vi "LC-MISDK_UserCalibration.vi"() -> ()   [LabVIEW 2015]
uses:
  C:/Users/e09031/Documents/GMA/LC-160/Labview/Sample_LC-MISDK/LC-MISDK.dll
  LC-MISDK.dll
panel:
  in  "タイムスタンプ":timestamp
  out "CalError":dbl
  out "error out":errorcluster caption="エラー出力"
  out "ErrorCode":dbl
  in  "Before_B 2":bool
  in  "Before_G 2":bool
  in  "Before_R 2":bool
  in  "Before_W 2":bool
  in  "After_B":T1
  in  "After_G":T2
  in  "After_R":T3
  in  "After_W":T4
  in  "Before_B":T5
  in  "Before_G":T6
  in  "Before_R":T7
  in  "Before_W":T8
  out "Error Message":string
  in  "EXIT":bool
  in  "Calib":bool
  in  "ID":string
  in  "Color Space":T9(ring)
  in  "Calib.Ch":T10(ring)
  in  "Type of Calibration":enum32{"Single-Point", "RGB", "WRGB"}(radio)
  # "Value before Calibration"
  # "Value after Calibration"
  # "X"
  # "Y"
  # "Z"
  # "X"
  # "Y"
  # "Z"
  # "White"
  # "White"
  # "Red"
  # "Red"
  # "Green"
  # "Green"
  # "Blue"
  # "Blue"
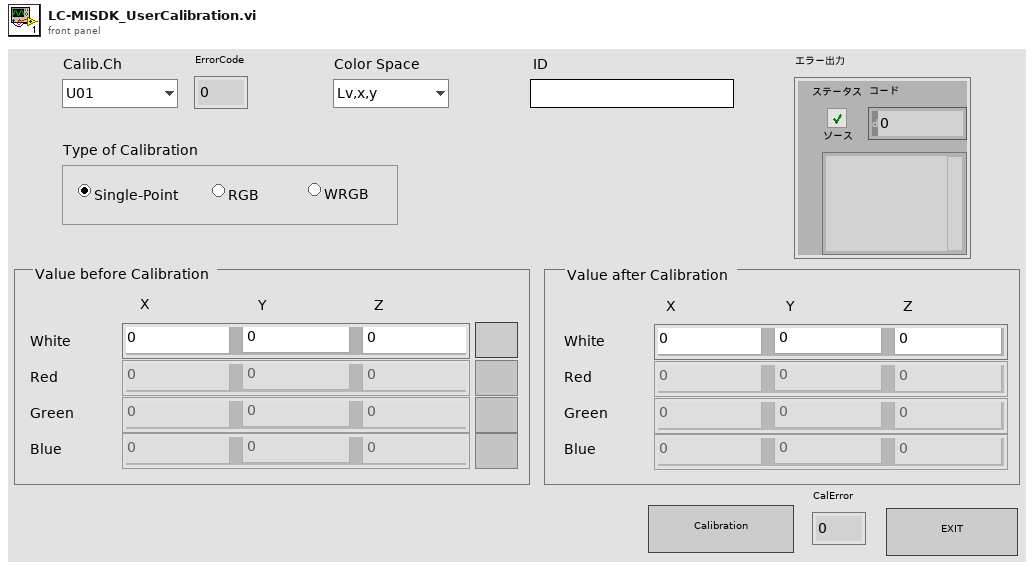
[diagram p1: front panel]
types:
  T1 = cluster{"After_B1":dbl, "After_B2":dbl, "After_B3":dbl}
  T2 = cluster{"After_G1":dbl, "After_G2":dbl, "After_G3":dbl}
  T3 = cluster{"After_R1":dbl, "After_R2":dbl, "After_R3":dbl}
  T4 = cluster{"After_W1":dbl, "After_W2":dbl, "After_W3":dbl}
  T5 = cluster{"before_B1":dbl, "Before_B2":dbl, "Before_B3":dbl}
  T6 = cluster{"before_G1":dbl, "Before_G2":dbl, "Before_G3":dbl}
  T7 = cluster{"before_R1":dbl, "Before_R2":dbl, "Before_R3":dbl}
  T8 = cluster{"before_W1":dbl, "Before_W2":dbl, "Before_W3":dbl}
  T9 = enum16{"Lv,x,y", "Lv,u',v'", "Lv,Tcp,duv", "X,Y,Z", "Lv,λd,Pe"}
  T10 = enum16{"U01", "U02", "U03", "U04", "U05", "U06", "U07", "U08", "U09", "U10"}
  T11 = cluster{"get_Item":dbl, "get_Item":dbl, "get_Item":dbl}
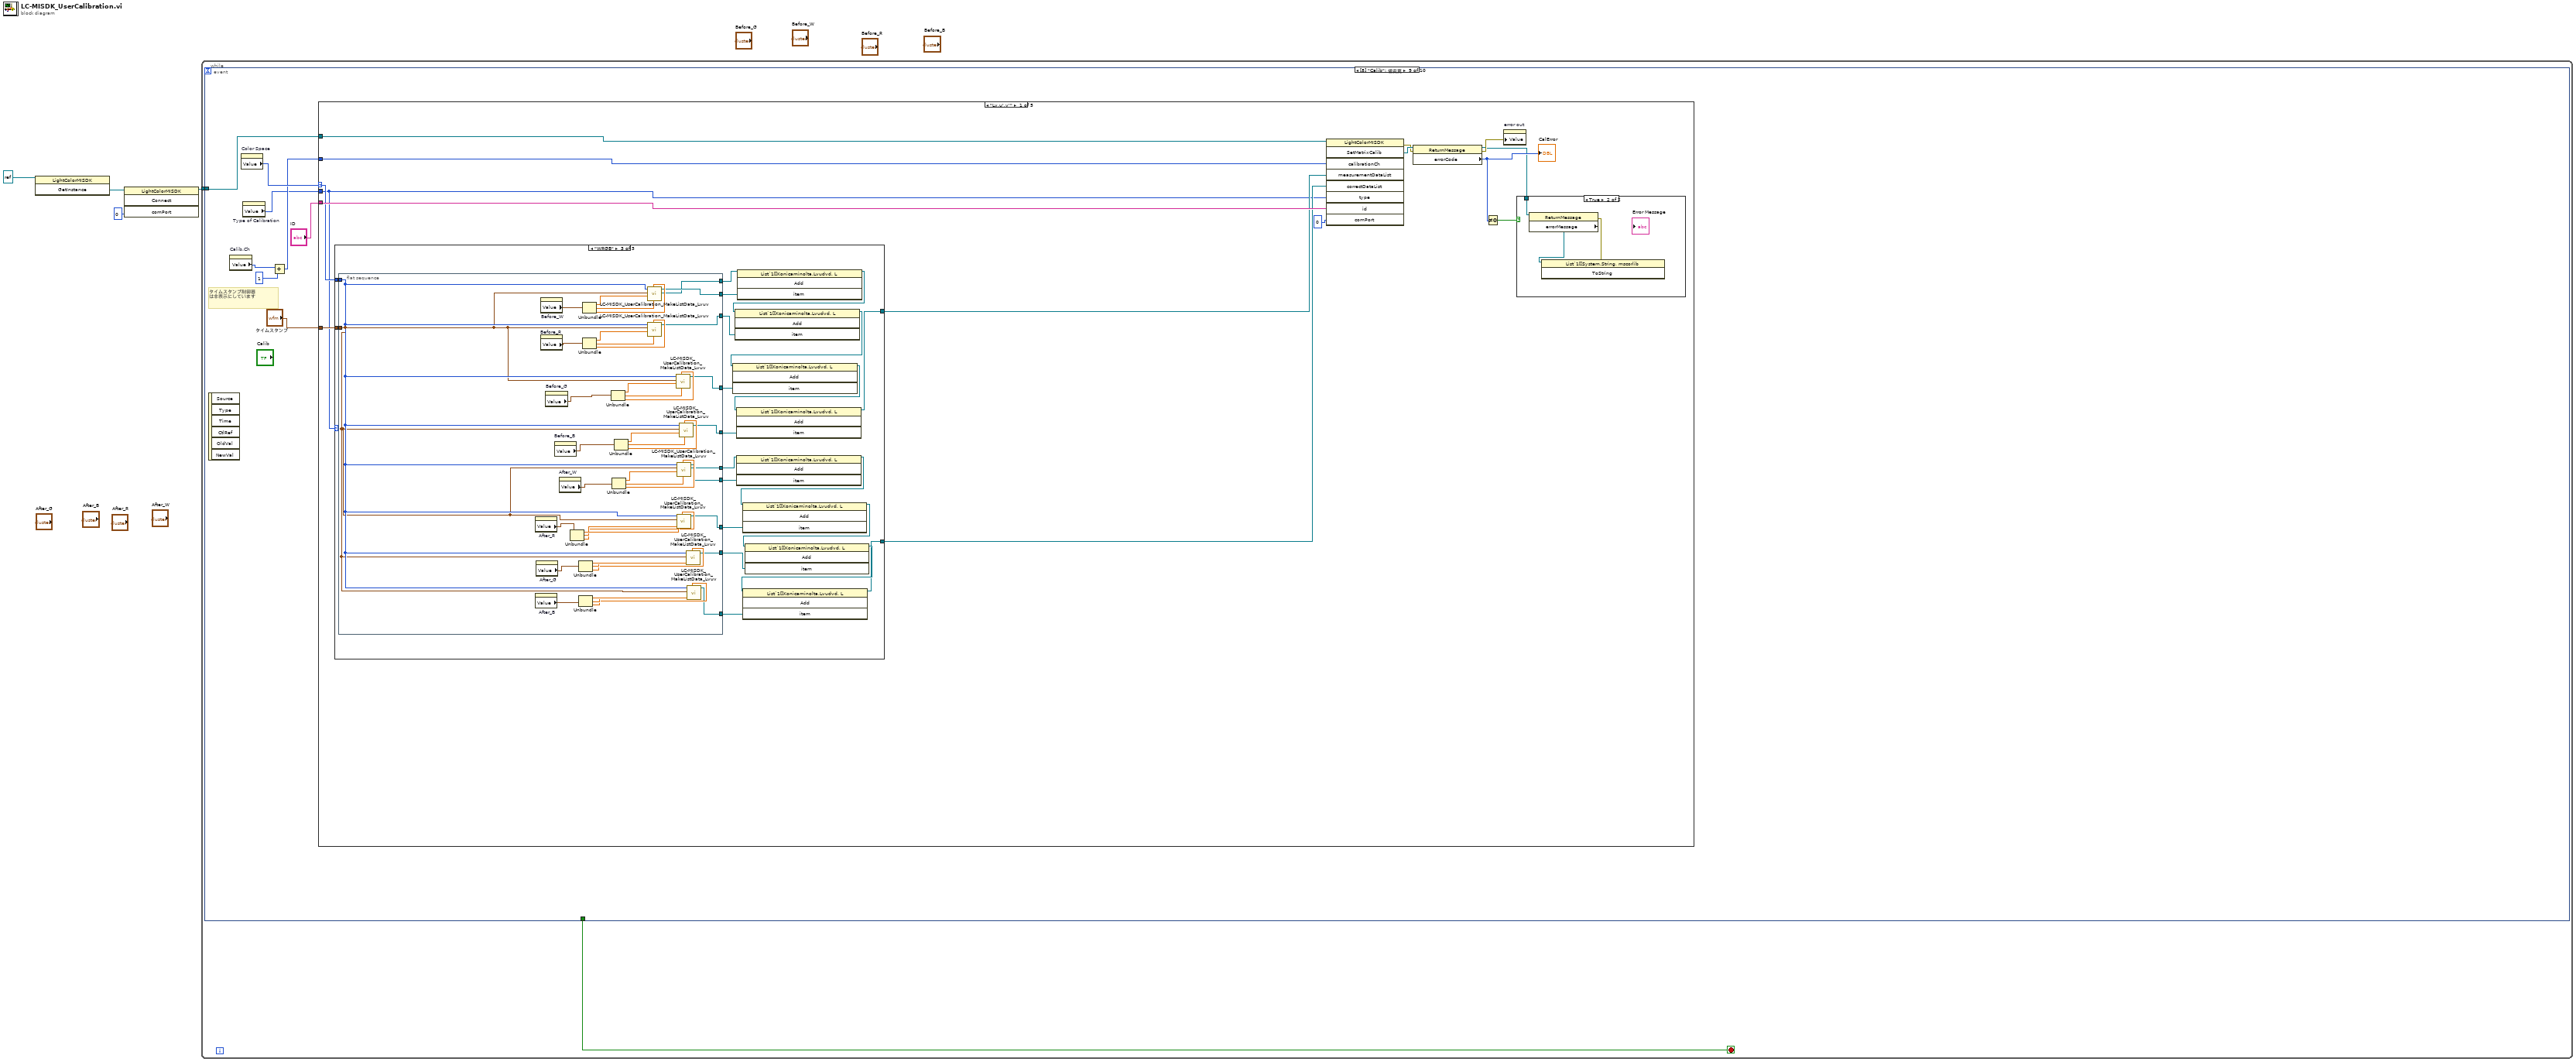
[diagram p0: block diagram]
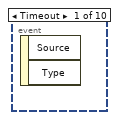
[diagram p2: hidden frame]
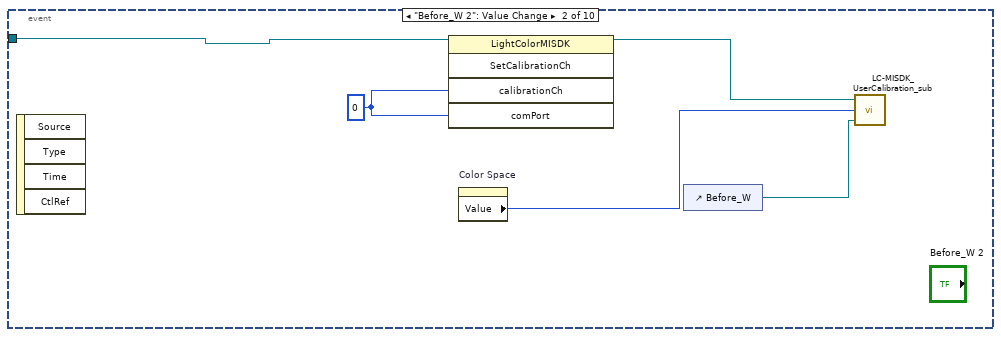
[diagram p3: hidden frame]
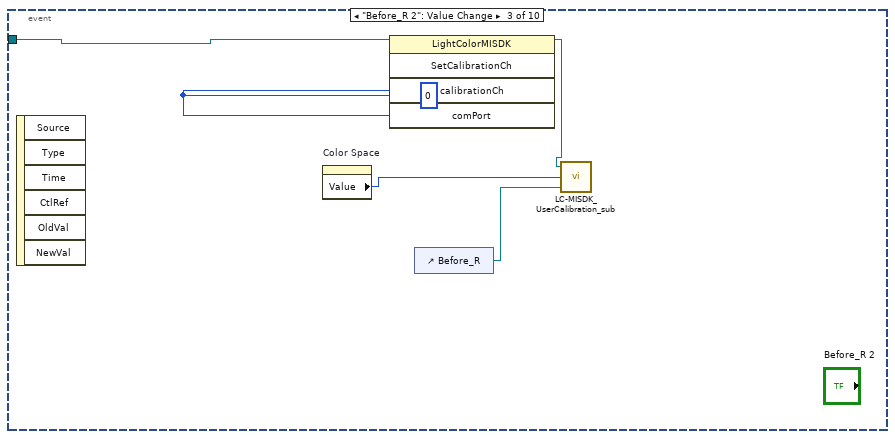
[diagram p4: hidden frame]
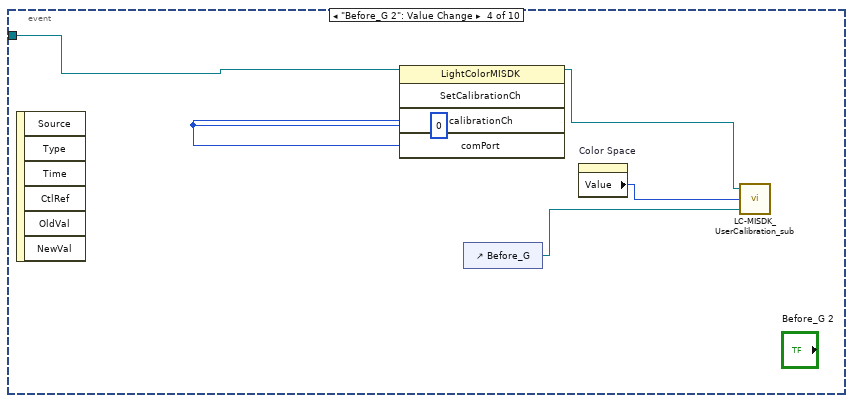
[diagram p5: hidden frame]
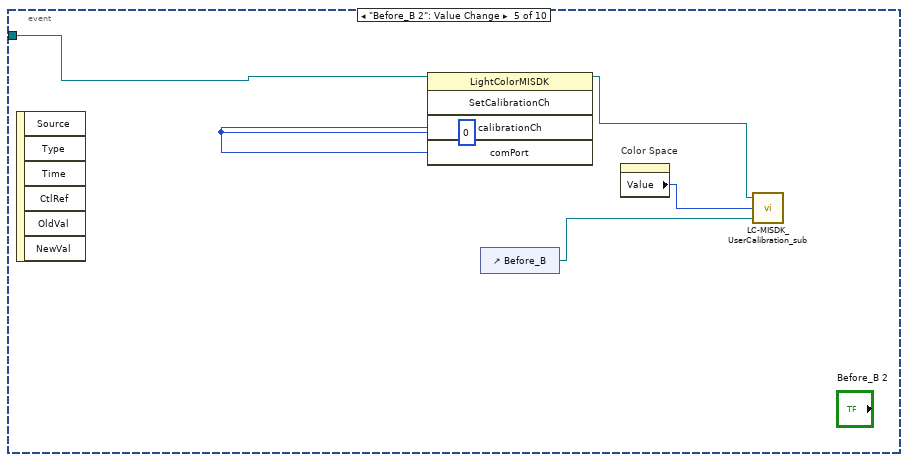
[diagram p6: hidden frame]
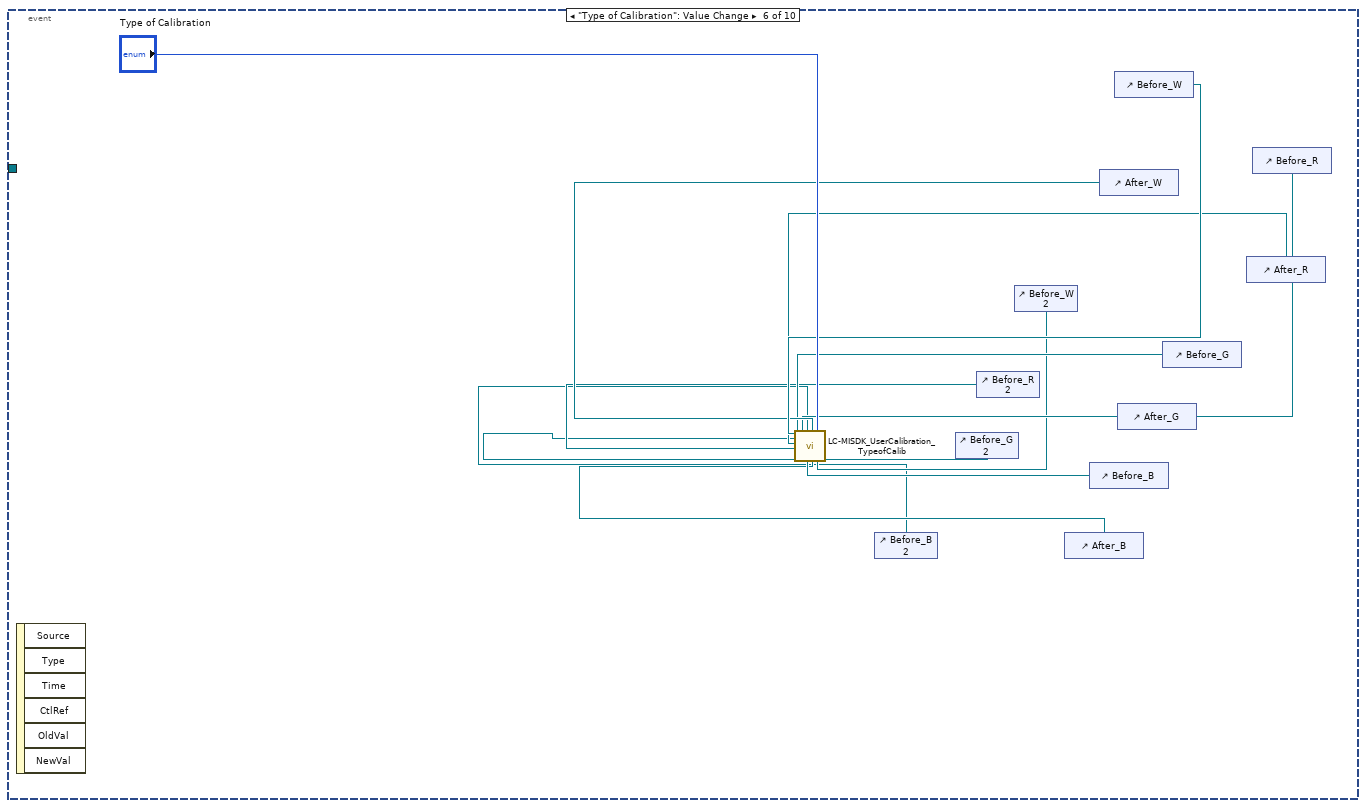
[diagram p7: hidden frame]
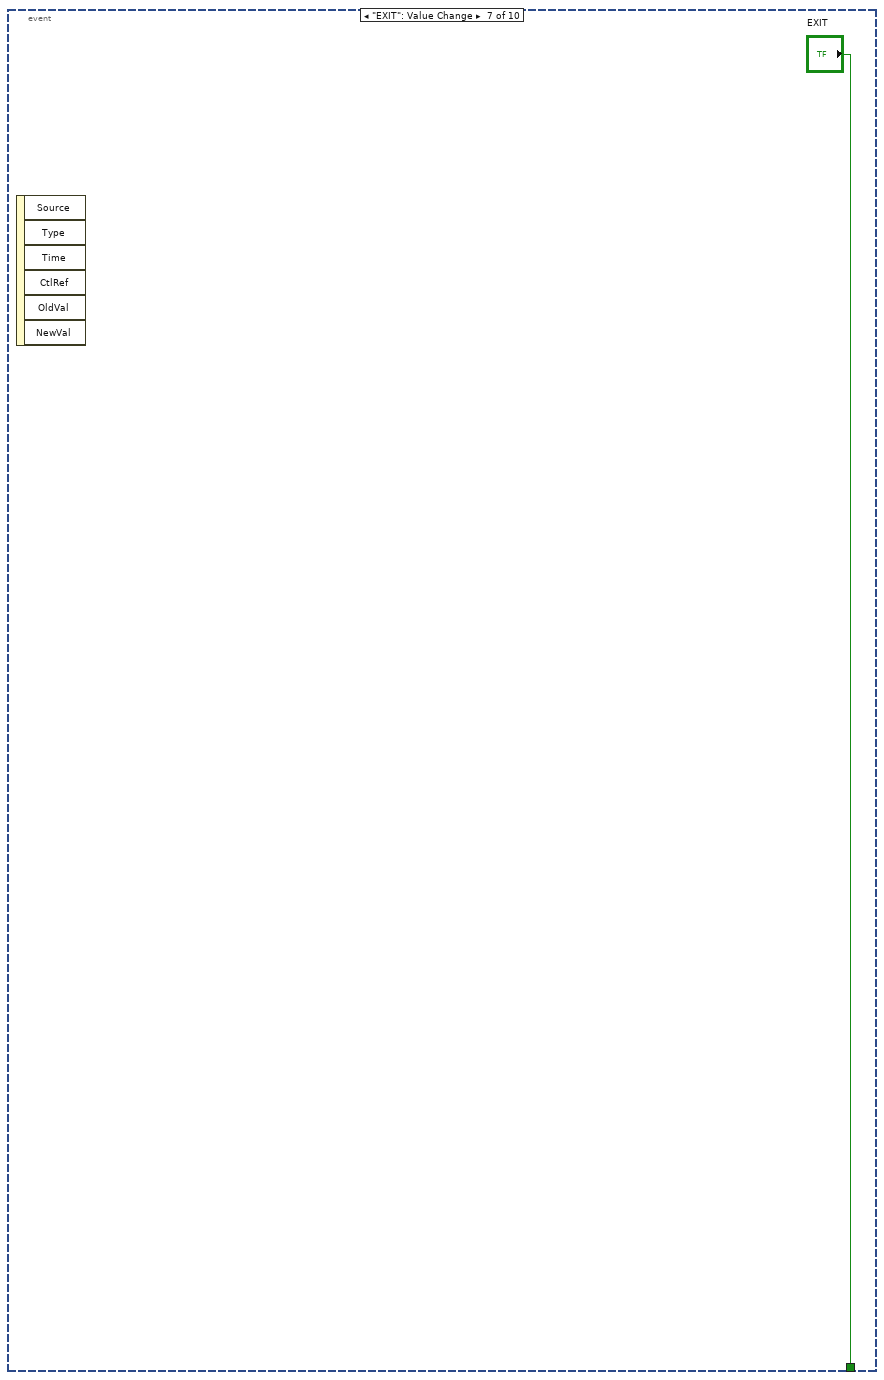
[diagram p8: hidden frame]
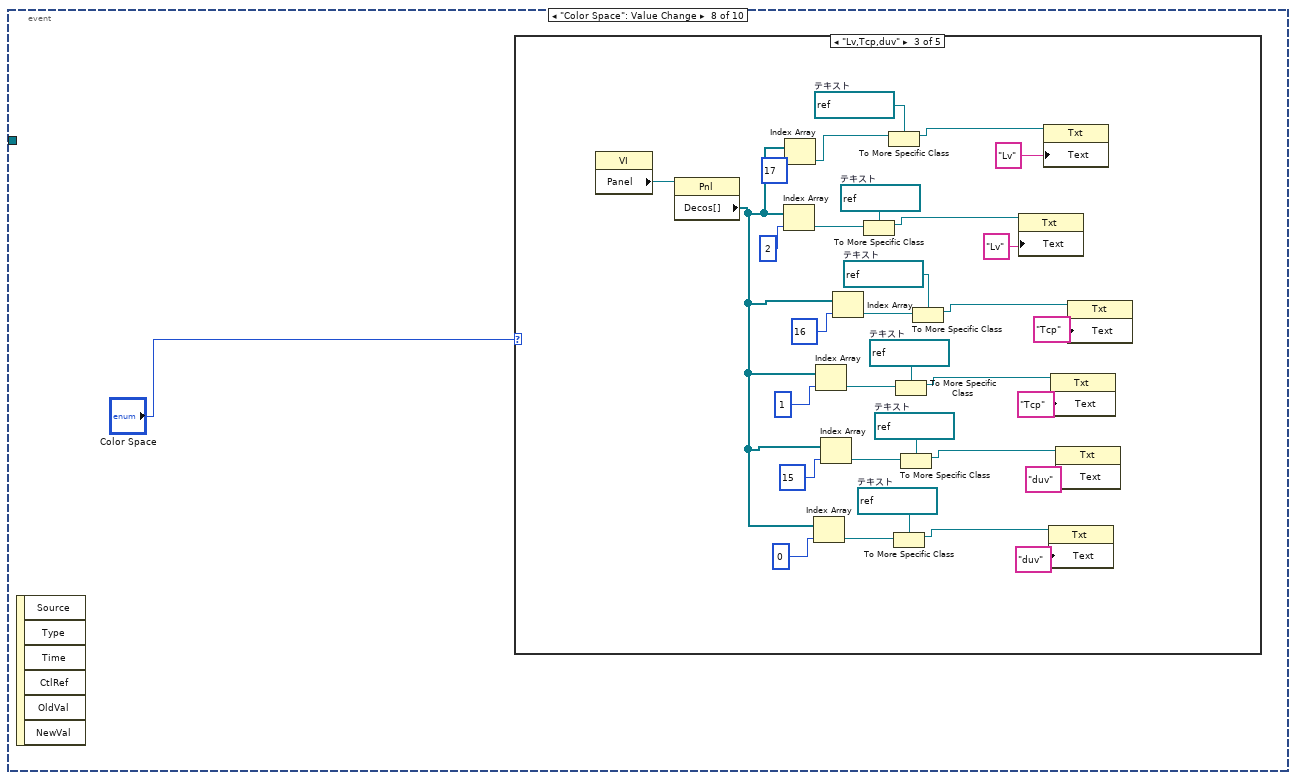
[diagram p9: hidden frame]
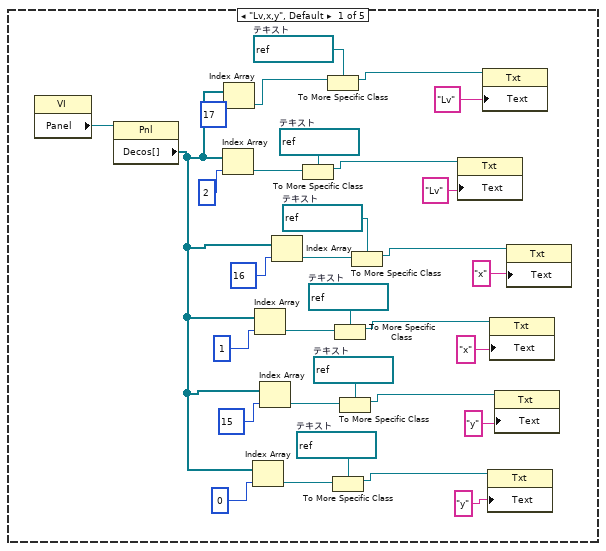
[diagram p10: hidden frame]
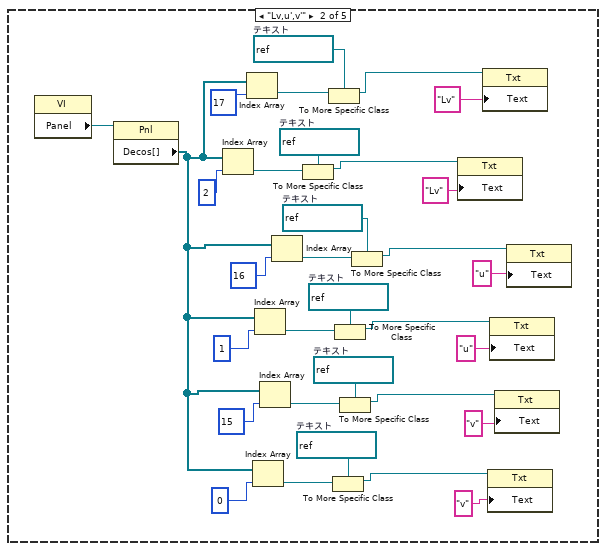
[diagram p11: hidden frame]
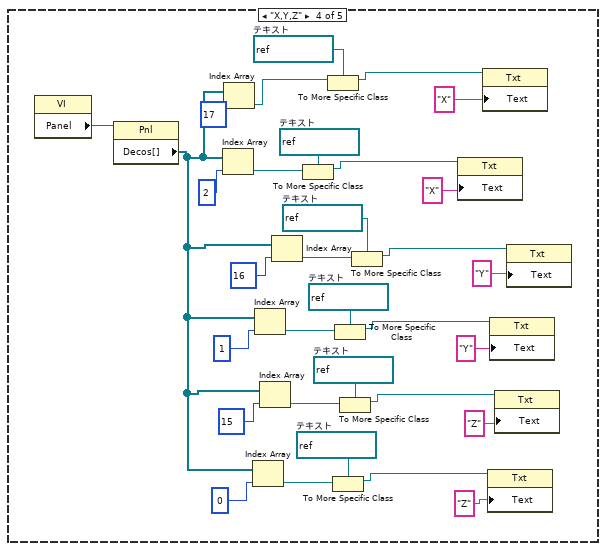
[diagram p12: hidden frame]
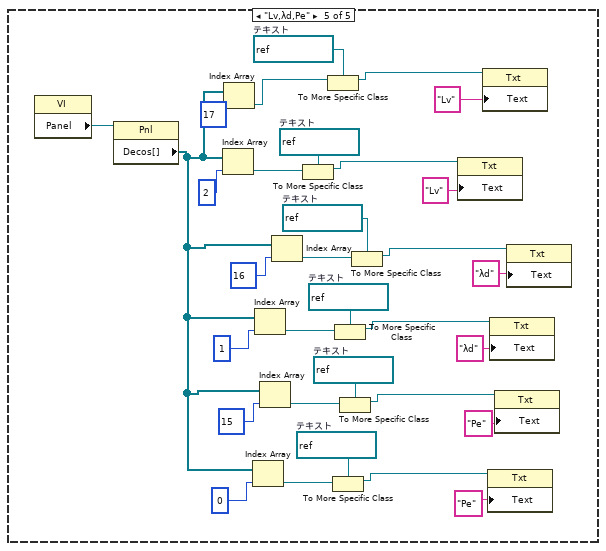
[diagram p13: hidden frame]
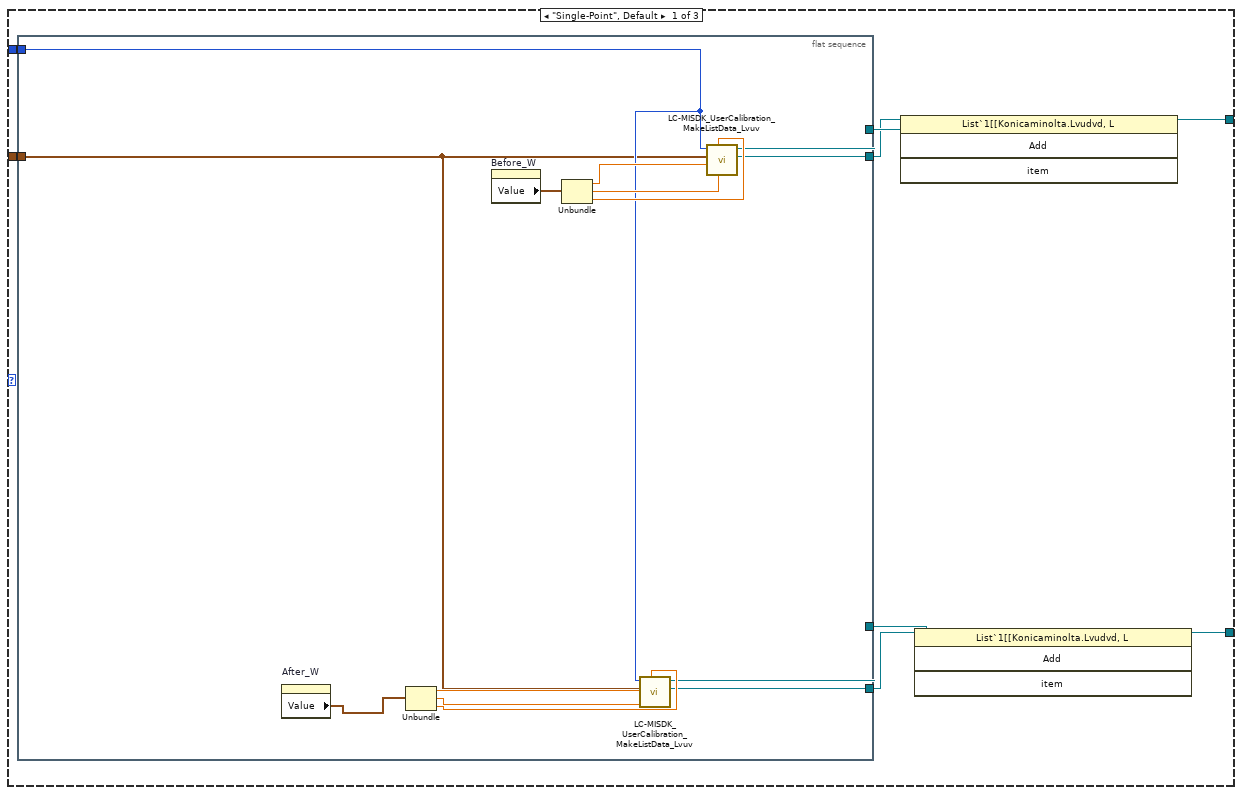
[diagram p15: hidden frame]
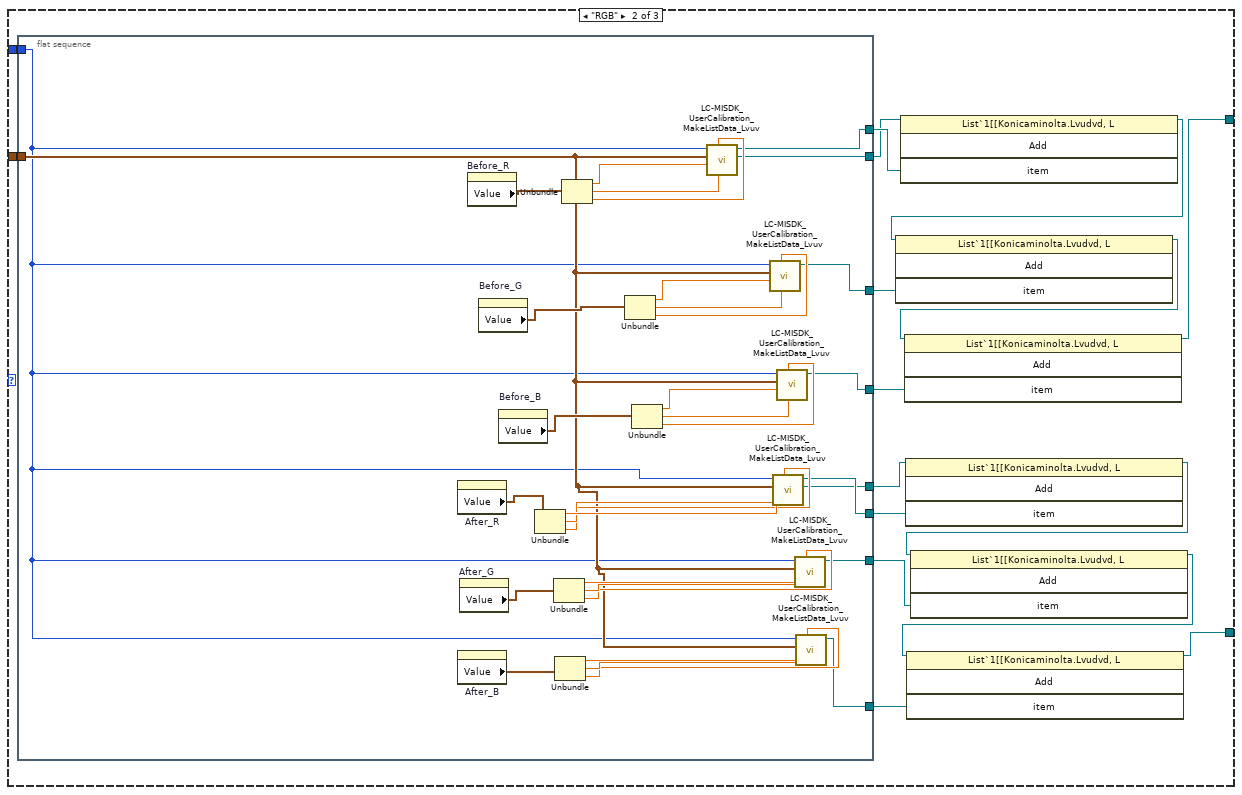
[diagram p16: hidden frame]
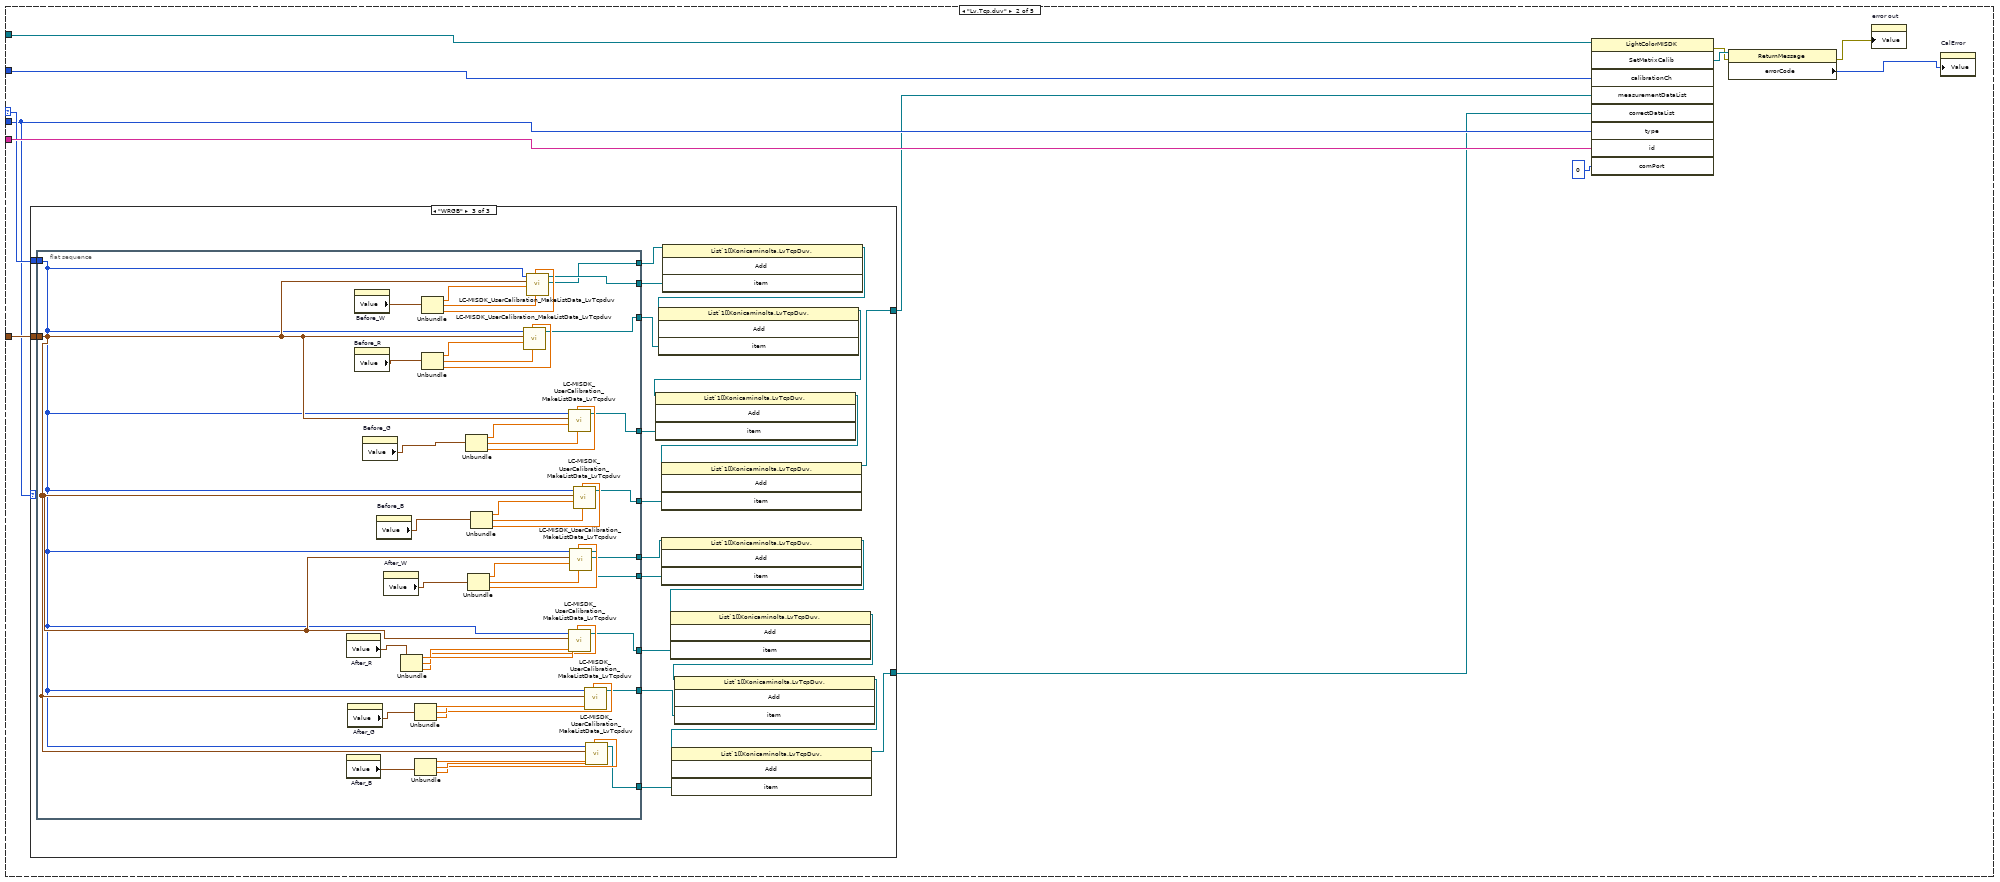
[diagram p17: hidden frame]
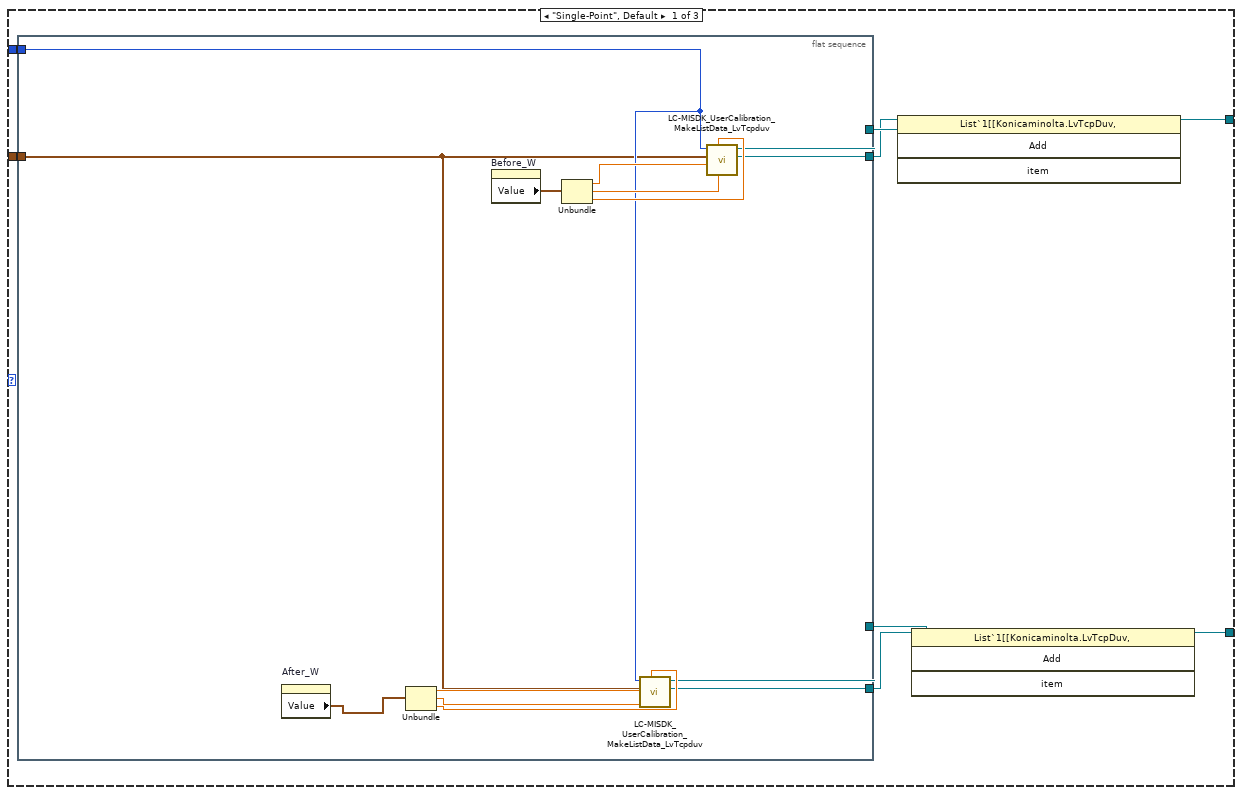
[diagram p18: hidden frame]
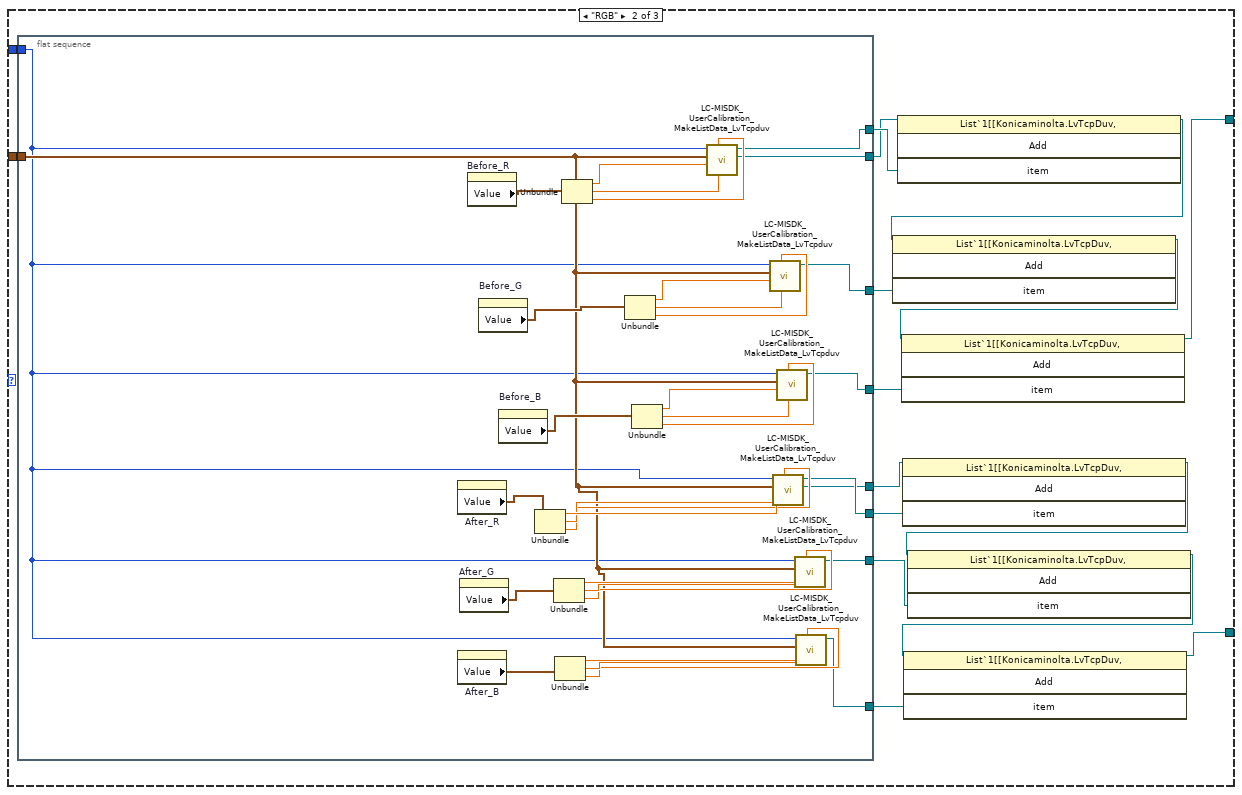
[diagram p19: hidden frame]
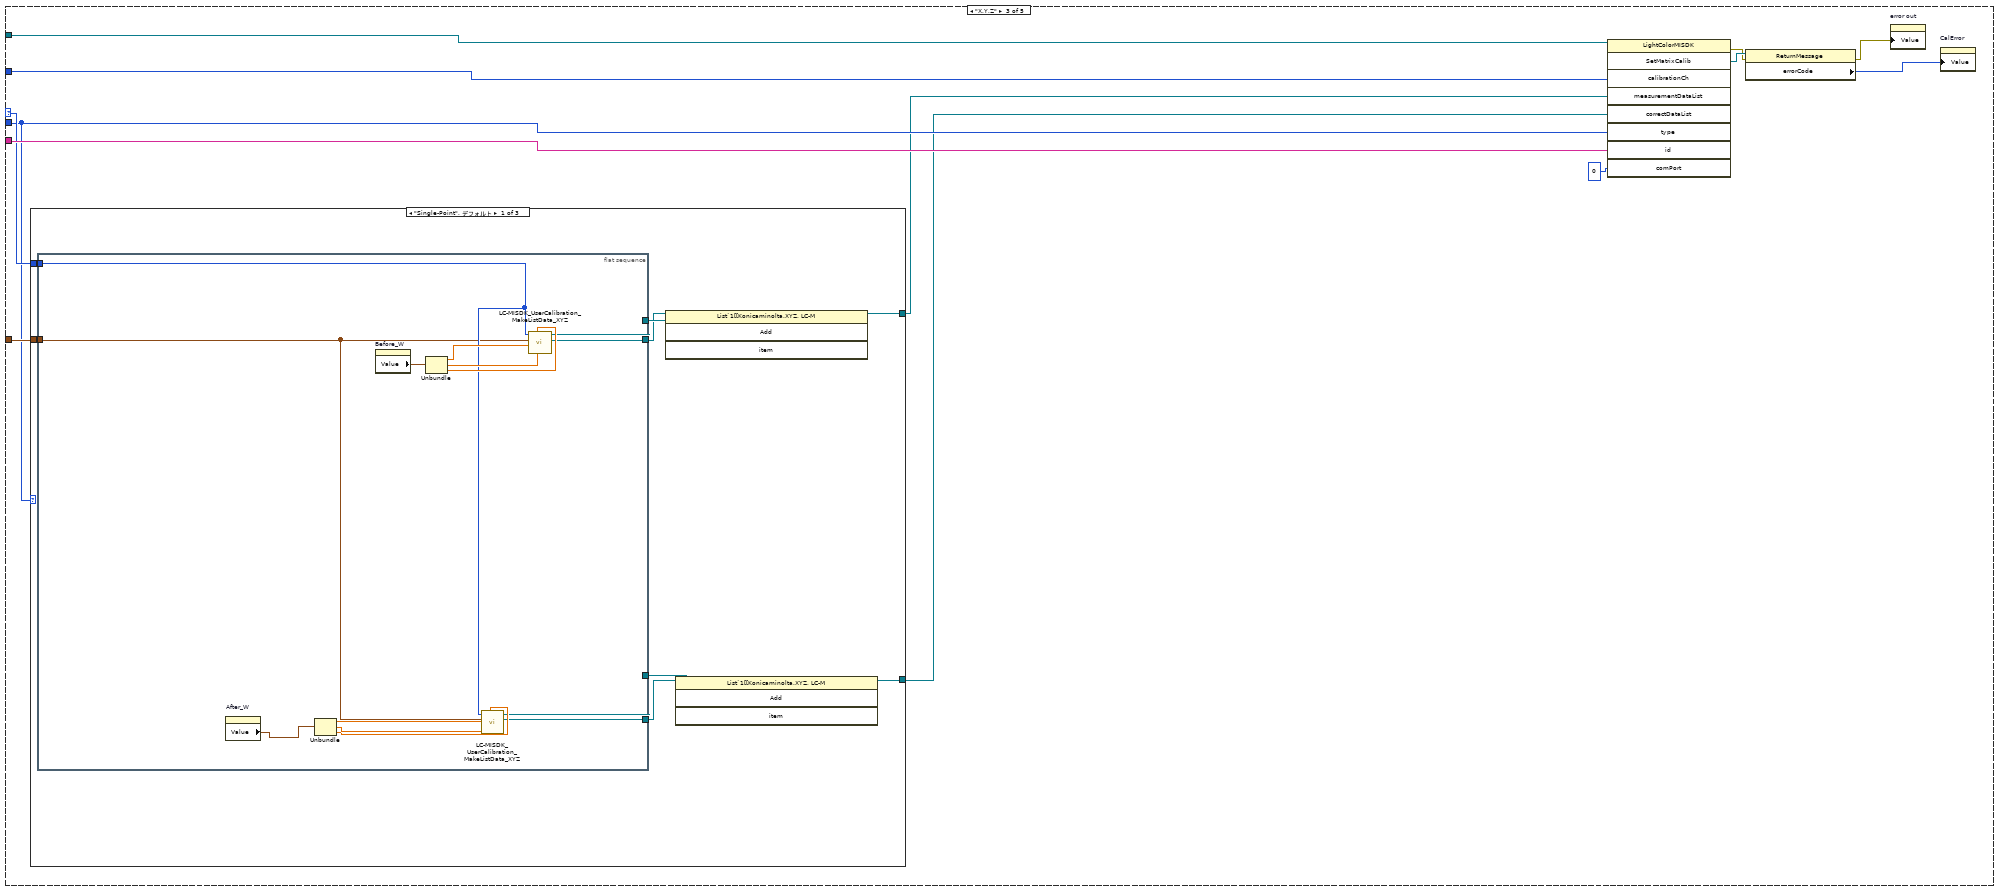
[diagram p20: hidden frame]
diagram:
  n1 = invoke on="インボークノード" class="LightColorMISDK" method="GetInstance"(reference=refnum<k24> refnum ("リファレンス出力")) -> ("GetInstance"=w3:refnum<k24>)  [unwired: 2 in, 2 out]
  n2 = invoke on="インボークノード" class="LightColorMISDK" method="Connect"(reference=w3, "comPort"=0) -> (reference out=w1:refnum<k24>)  [unwired: 2 in, 3 out]
  n3 = while {
    tunnel: w1 -> [w6]
    stop <- w5 stop-if-true
    n4 = event shown="[8] \"Calib\": 値変更" {
      selector: _ -> [_ _ _ _ _ _ _ _ _ _]
      dyn-events: _ -> [_ _ _ _ _ _ _ _ _ _]
      timeout: _ -> [_ _ _ _ _ _ _ _ _ _]
      tunnel: w6 -> [_ w10 w13 w18 w23 _ _ _ w207 w966]
      tunnel: [_ _ _ _ _ _ "EXIT" _ _ _] -> w5
      event Timeout {
        n5 = event-data() -> ()  [unwired: 1 in, 2 out]
      }
      event "Before_W 2": Value Change {
        w8 = 0
        n6 = event-data() -> ()  [unwired: 1 in, 4 out]
        n7 = invoke on="インボークノード" class="LightColorMISDK" method="SetCalibrationCh"(reference=w10, "calibrationCh"=w8, "comPort"=w8) -> (reference out=w9:refnum<k24>)  [unwired: 2 in, 4 out]
        n8 = property on="Color Space" class="Enum （指定）"() -> ("Value"=w7:T9)  [unwired: 2 in, 2 out]
        n9 = control-ref of="Before_W"() -> (w11:refnum<vi>)
        n10 = call "LC-MISDK_UserCalibration_sub.vi"(".NET refnum入力"=w9, "Color Space"=w7, "Clust refnum"=w11) -> ()  [unwired: 5 in]
      }
      event "Before_R 2": Value Change {
        w15 = 0
        n11 = event-data() -> ()  [unwired: 1 in, 6 out]
        n12 = property on="Color Space" class="Enum （指定）"() -> ("Value"=w12:T9)  [unwired: 2 in, 2 out]
        n13 = invoke on="インボークノード" class="LightColorMISDK" method="SetCalibrationCh"(reference=w13, "calibrationCh"=w15, "comPort"=w15) -> (reference out=w14:refnum<k24>)  [unwired: 2 in, 4 out]
        n14 = control-ref of="Before_R"() -> (w16:refnum<vi>)
        n15 = call "LC-MISDK_UserCalibration_sub.vi"(".NET refnum入力"=w14, "Color Space"=w12, "Clust refnum"=w16) -> ()  [unwired: 5 in]
      }
      event "Before_G 2": Value Change {
        w20 = 0
        n16 = event-data() -> ()  [unwired: 1 in, 6 out]
        n17 = invoke on="インボークノード" class="LightColorMISDK" method="SetCalibrationCh"(reference=w18, "calibrationCh"=w20, "comPort"=w20) -> (reference out=w19:refnum<k24>)  [unwired: 2 in, 4 out]
        n18 = control-ref of="Before_G"() -> (w21:refnum<vi>)
        n19 = property on="Color Space" class="Enum （指定）"() -> ("Value"=w17:T9)  [unwired: 2 in, 2 out]
        n20 = call "LC-MISDK_UserCalibration_sub.vi"(".NET refnum入力"=w19, "Color Space"=w17, "Clust refnum"=w21) -> ()  [unwired: 5 in]
      }
      event "Before_B 2": Value Change {
        w25 = 0
        n21 = event-data() -> ()  [unwired: 1 in, 6 out]
        n22 = invoke on="インボークノード" class="LightColorMISDK" method="SetCalibrationCh"(reference=w23, "calibrationCh"=w25, "comPort"=w25) -> (reference out=w24:refnum<k24>)  [unwired: 2 in, 4 out]
        n23 = control-ref of="Before_B"() -> (w26:refnum<vi>)
        n24 = property on="Color Space" class="Enum （指定）"() -> ("Value"=w22:T9)  [unwired: 2 in, 2 out]
        n25 = call "LC-MISDK_UserCalibration_sub.vi"(".NET refnum入力"=w24, "Color Space"=w22, "Clust refnum"=w26) -> ()  [unwired: 5 in]
      }
      event "Type of Calibration": Value Change {
        n26 = event-data() -> ()  [unwired: 1 in, 6 out]
        n27 = control-ref of="Before_B 2"() -> (w27:refnum<vi>)
        n28 = control-ref of="Before_G 2"() -> (w28:refnum<vi>)
        n29 = control-ref of="Before_R 2"() -> (w29:refnum<vi>)
        n30 = control-ref of="Before_W 2"() -> (w30:refnum<vi>)
        n31 = control-ref of="After_B"() -> (w31:refnum<vi>)
        n32 = control-ref of="Before_B"() -> (w32:refnum<vi>)
        n33 = control-ref of="After_W"() -> (w37:refnum<vi>)
        n34 = control-ref of="Before_W"() -> (w38:refnum<vi>)
        n35 = control-ref of="After_G"() -> (w33:refnum<vi>)
        n36 = control-ref of="Before_G"() -> (w34:refnum<vi>)
        n37 = control-ref of="After_R"() -> (w35:refnum<vi>)
        n38 = control-ref of="Before_R"() -> (w36:refnum<vi>)
        n39 = call "LC-MISDK_UserCalibration_TypeofCalib.vi"("Cluster入力"=w38, "Bool refnum 3"=w28, "Clust refnum 4"=w35, "Bool refnum 2"=w29, "Clust refnum 5"=w34, "Clust refnum 3"=w36, "Clust refnum 6"=w33, "Bool refnum 4"=w27, "Clust refnum 7"=w32, "Clust refnum入力"=w37, "Clust refnum 8"=w31, "Type of Calibration"="Type of Calibration", "Bool refnum"=w30) -> ()  [unwired: 7 in]
      }
      event "EXIT": Value Change {
        n40 = event-data() -> ()  [unwired: 1 in, 6 out]
      }
      event "Color Space": Value Change {
        n41 = event-data() -> ()  [unwired: 1 in, 6 out]
        n42 = case shown="\"Lv,Tcp,duv\"" "Color Space" {
          frame "Lv,x,y", Default {
            w45 = refnum<vi> refnum  # テキスト
            w50 = refnum<vi> refnum  # テキスト
            w53 = refnum<vi> refnum  # テキスト
            w60 = refnum<vi> refnum  # テキスト
            w65 = refnum<vi> refnum  # テキスト
            w70 = refnum<vi> refnum  # テキスト
            n43 = property class="VI"() -> ("Panel"=w73:refnum<vi>)  [unwired: 2 in, 2 out]
            n44 = property class="Pnl"(reference=w73) -> ("Decos[]"=w42:refnum<vi>[])  [unwired: 1 in, 2 out]
            n45 = Index Array(array=w42, index=2) -> (element=w72:refnum<vi>)
            n46 = Index Array(array=w42, index=17) -> (element=w55:refnum<vi>)
            n47 = Index Array(array=w42, index=0) -> (element=w62:refnum<vi>)
            n48 = Index Array(array=w42, index=1) -> (element=w67:refnum<vi>)
            n49 = Index Array(array=w42, index=15) -> (element=w47:refnum<vi>)
            n50 = Index Array(array=w42, index=16) -> (element=w52:refnum<vi>)
            n51 = To More Specific Class(target class=w70, reference=w72) -> (specific class reference=w71:refnum<vi>)  [unwired: 1 in, 1 out]
            n52 = To More Specific Class(target class=w53, reference=w55) -> (specific class reference=w57:refnum<vi>)  [unwired: 1 in, 1 out]
            n53 = To More Specific Class(target class=w60, reference=w62) -> (specific class reference=w61:refnum<vi>)  [unwired: 1 in, 1 out]
            n54 = To More Specific Class(target class=w65, reference=w67) -> (specific class reference=w66:refnum<vi>)  [unwired: 1 in, 1 out]
            n55 = To More Specific Class(target class=w45, reference=w47) -> (specific class reference=w46:refnum<vi>)  [unwired: 1 in, 1 out]
            n56 = To More Specific Class(target class=w50, reference=w52) -> (specific class reference=w51:refnum<vi>)  [unwired: 1 in, 1 out]
            n57 = property class="Txt"(reference=w71, "Text"="Lv") -> ()  [unwired: 1 in, 2 out]
            n58 = property class="Txt"(reference=w57, "Text"="Lv") -> ()  [unwired: 1 in, 2 out]
            n59 = property class="Txt"(reference=w61, "Text"="y") -> ()  [unwired: 1 in, 2 out]
            n60 = property class="Txt"(reference=w66, "Text"="x") -> ()  [unwired: 1 in, 2 out]
            n61 = property class="Txt"(reference=w46, "Text"="y") -> ()  [unwired: 1 in, 2 out]
            n62 = property class="Txt"(reference=w51, "Text"="x") -> ()  [unwired: 1 in, 2 out]
          }
          frame "Lv,u',v'" {
            w77 = refnum<vi> refnum  # テキスト
            w82 = refnum<vi> refnum  # テキスト
            w85 = refnum<vi> refnum  # テキスト
            w92 = refnum<vi> refnum  # テキスト
            w97 = refnum<vi> refnum  # テキスト
            w102 = refnum<vi> refnum  # テキスト
            n63 = property class="VI"() -> ("Panel"=w105:refnum<vi>)  [unwired: 2 in, 2 out]
            n64 = property class="Pnl"(reference=w105) -> ("Decos[]"=w74:refnum<vi>[])  [unwired: 1 in, 2 out]
            n65 = Index Array(array=w74, index=2) -> (element=w104:refnum<vi>)
            n66 = Index Array(array=w74, index=17) -> (element=w87:refnum<vi>)
            n67 = Index Array(array=w74, index=0) -> (element=w94:refnum<vi>)
            n68 = Index Array(array=w74, index=1) -> (element=w99:refnum<vi>)
            n69 = Index Array(array=w74, index=15) -> (element=w79:refnum<vi>)
            n70 = Index Array(array=w74, index=16) -> (element=w84:refnum<vi>)
            n71 = To More Specific Class(target class=w102, reference=w104) -> (specific class reference=w103:refnum<vi>)  [unwired: 1 in, 1 out]
            n72 = To More Specific Class(target class=w85, reference=w87) -> (specific class reference=w89:refnum<vi>)  [unwired: 1 in, 1 out]
            n73 = To More Specific Class(target class=w92, reference=w94) -> (specific class reference=w93:refnum<vi>)  [unwired: 1 in, 1 out]
            n74 = To More Specific Class(target class=w97, reference=w99) -> (specific class reference=w98:refnum<vi>)  [unwired: 1 in, 1 out]
            n75 = To More Specific Class(target class=w77, reference=w79) -> (specific class reference=w78:refnum<vi>)  [unwired: 1 in, 1 out]
            n76 = To More Specific Class(target class=w82, reference=w84) -> (specific class reference=w83:refnum<vi>)  [unwired: 1 in, 1 out]
            n77 = property class="Txt"(reference=w103, "Text"="Lv") -> ()  [unwired: 1 in, 2 out]
            n78 = property class="Txt"(reference=w89, "Text"="Lv") -> ()  [unwired: 1 in, 2 out]
            n79 = property class="Txt"(reference=w93, "Text"="v") -> ()  [unwired: 1 in, 2 out]
            n80 = property class="Txt"(reference=w98, "Text"="u") -> ()  [unwired: 1 in, 2 out]
            n81 = property class="Txt"(reference=w78, "Text"="v") -> ()  [unwired: 1 in, 2 out]
            n82 = property class="Txt"(reference=w83, "Text"="u") -> ()  [unwired: 1 in, 2 out]
          }
          frame "Lv,Tcp,duv" {
            w109 = refnum<vi> refnum  # テキスト
            w114 = refnum<vi> refnum  # テキスト
            w117 = refnum<vi> refnum  # テキスト
            w124 = refnum<vi> refnum  # テキスト
            w129 = refnum<vi> refnum  # テキスト
            w134 = refnum<vi> refnum  # テキスト
            n83 = property class="VI"() -> ("Panel"=w137:refnum<vi>)  [unwired: 2 in, 2 out]
            n84 = property class="Pnl"(reference=w137) -> ("Decos[]"=w106:refnum<vi>[])  [unwired: 1 in, 2 out]
            n85 = Index Array(array=w106, index=2) -> (element=w136:refnum<vi>)
            n86 = Index Array(array=w106, index=17) -> (element=w119:refnum<vi>)
            n87 = Index Array(array=w106, index=0) -> (element=w126:refnum<vi>)
            n88 = Index Array(array=w106, index=1) -> (element=w131:refnum<vi>)
            n89 = Index Array(array=w106, index=15) -> (element=w111:refnum<vi>)
            n90 = Index Array(array=w106, index=16) -> (element=w116:refnum<vi>)
            n91 = To More Specific Class(target class=w134, reference=w136) -> (specific class reference=w135:refnum<vi>)  [unwired: 1 in, 1 out]
            n92 = To More Specific Class(target class=w117, reference=w119) -> (specific class reference=w121:refnum<vi>)  [unwired: 1 in, 1 out]
            n93 = To More Specific Class(target class=w124, reference=w126) -> (specific class reference=w125:refnum<vi>)  [unwired: 1 in, 1 out]
            n94 = To More Specific Class(target class=w129, reference=w131) -> (specific class reference=w130:refnum<vi>)  [unwired: 1 in, 1 out]
            n95 = To More Specific Class(target class=w109, reference=w111) -> (specific class reference=w110:refnum<vi>)  [unwired: 1 in, 1 out]
            n96 = To More Specific Class(target class=w114, reference=w116) -> (specific class reference=w115:refnum<vi>)  [unwired: 1 in, 1 out]
            n97 = property class="Txt"(reference=w135, "Text"="Lv") -> ()  [unwired: 1 in, 2 out]
            n98 = property class="Txt"(reference=w121, "Text"="Lv") -> ()  [unwired: 1 in, 2 out]
            n99 = property class="Txt"(reference=w125, "Text"="duv") -> ()  [unwired: 1 in, 2 out]
            n100 = property class="Txt"(reference=w130, "Text"="Tcp") -> ()  [unwired: 1 in, 2 out]
            n101 = property class="Txt"(reference=w110, "Text"="duv") -> ()  [unwired: 1 in, 2 out]
            n102 = property class="Txt"(reference=w115, "Text"="Tcp") -> ()  [unwired: 1 in, 2 out]
          }
          frame "X,Y,Z" {
            w141 = refnum<vi> refnum  # テキスト
            w146 = refnum<vi> refnum  # テキスト
            w149 = refnum<vi> refnum  # テキスト
            w156 = refnum<vi> refnum  # テキスト
            w161 = refnum<vi> refnum  # テキスト
            w166 = refnum<vi> refnum  # テキスト
            n103 = property class="VI"() -> ("Panel"=w169:refnum<vi>)  [unwired: 2 in, 2 out]
            n104 = property class="Pnl"(reference=w169) -> ("Decos[]"=w138:refnum<vi>[])  [unwired: 1 in, 2 out]
            n105 = Index Array(array=w138, index=2) -> (element=w168:refnum<vi>)
            n106 = Index Array(array=w138, index=17) -> (element=w151:refnum<vi>)
            n107 = Index Array(array=w138, index=0) -> (element=w158:refnum<vi>)
            n108 = Index Array(array=w138, index=1) -> (element=w163:refnum<vi>)
            n109 = Index Array(array=w138, index=15) -> (element=w143:refnum<vi>)
            n110 = Index Array(array=w138, index=16) -> (element=w148:refnum<vi>)
            n111 = To More Specific Class(target class=w166, reference=w168) -> (specific class reference=w167:refnum<vi>)  [unwired: 1 in, 1 out]
            n112 = To More Specific Class(target class=w149, reference=w151) -> (specific class reference=w153:refnum<vi>)  [unwired: 1 in, 1 out]
            n113 = To More Specific Class(target class=w156, reference=w158) -> (specific class reference=w157:refnum<vi>)  [unwired: 1 in, 1 out]
            n114 = To More Specific Class(target class=w161, reference=w163) -> (specific class reference=w162:refnum<vi>)  [unwired: 1 in, 1 out]
            n115 = To More Specific Class(target class=w141, reference=w143) -> (specific class reference=w142:refnum<vi>)  [unwired: 1 in, 1 out]
            n116 = To More Specific Class(target class=w146, reference=w148) -> (specific class reference=w147:refnum<vi>)  [unwired: 1 in, 1 out]
            n117 = property class="Txt"(reference=w167, "Text"="X") -> ()  [unwired: 1 in, 2 out]
            n118 = property class="Txt"(reference=w153, "Text"="X") -> ()  [unwired: 1 in, 2 out]
            n119 = property class="Txt"(reference=w157, "Text"="Z") -> ()  [unwired: 1 in, 2 out]
            n120 = property class="Txt"(reference=w162, "Text"="Y") -> ()  [unwired: 1 in, 2 out]
            n121 = property class="Txt"(reference=w142, "Text"="Z") -> ()  [unwired: 1 in, 2 out]
            n122 = property class="Txt"(reference=w147, "Text"="Y") -> ()  [unwired: 1 in, 2 out]
          }
          frame "Lv,λd,Pe" {
            w173 = refnum<vi> refnum  # テキスト
            w178 = refnum<vi> refnum  # テキスト
            w181 = refnum<vi> refnum  # テキスト
            w188 = refnum<vi> refnum  # テキスト
            w193 = refnum<vi> refnum  # テキスト
            w198 = refnum<vi> refnum  # テキスト
            n123 = property class="VI"() -> ("Panel"=w201:refnum<vi>)  [unwired: 2 in, 2 out]
            n124 = property class="Pnl"(reference=w201) -> ("Decos[]"=w170:refnum<vi>[])  [unwired: 1 in, 2 out]
            n125 = Index Array(array=w170, index=2) -> (element=w200:refnum<vi>)
            n126 = Index Array(array=w170, index=17) -> (element=w183:refnum<vi>)
            n127 = Index Array(array=w170, index=0) -> (element=w190:refnum<vi>)
            n128 = Index Array(array=w170, index=1) -> (element=w195:refnum<vi>)
            n129 = Index Array(array=w170, index=15) -> (element=w175:refnum<vi>)
            n130 = Index Array(array=w170, index=16) -> (element=w180:refnum<vi>)
            n131 = To More Specific Class(target class=w198, reference=w200) -> (specific class reference=w199:refnum<vi>)  [unwired: 1 in, 1 out]
            n132 = To More Specific Class(target class=w181, reference=w183) -> (specific class reference=w185:refnum<vi>)  [unwired: 1 in, 1 out]
            n133 = To More Specific Class(target class=w188, reference=w190) -> (specific class reference=w189:refnum<vi>)  [unwired: 1 in, 1 out]
            n134 = To More Specific Class(target class=w193, reference=w195) -> (specific class reference=w194:refnum<vi>)  [unwired: 1 in, 1 out]
            n135 = To More Specific Class(target class=w173, reference=w175) -> (specific class reference=w174:refnum<vi>)  [unwired: 1 in, 1 out]
            n136 = To More Specific Class(target class=w178, reference=w180) -> (specific class reference=w179:refnum<vi>)  [unwired: 1 in, 1 out]
            n137 = property class="Txt"(reference=w199, "Text"="Lv") -> ()  [unwired: 1 in, 2 out]
            n138 = property class="Txt"(reference=w185, "Text"="Lv") -> ()  [unwired: 1 in, 2 out]
            n139 = property class="Txt"(reference=w189, "Text"="Pe") -> ()  [unwired: 1 in, 2 out]
            n140 = property class="Txt"(reference=w194, "Text"="λd") -> ()  [unwired: 1 in, 2 out]
            n141 = property class="Txt"(reference=w174, "Text"="Pe") -> ()  [unwired: 1 in, 2 out]
            n142 = property class="Txt"(reference=w179, "Text"="λd") -> ()  [unwired: 1 in, 2 out]
          }
        }
      }
      event "Calib": Value Change {
        # "タイムスタンプ制御器\nは非表示にしています"
        n143 = event-data() -> ()  [unwired: 1 in, 6 out]
        n144 = property on="Calib.Ch" class="Enum （指定）"() -> ("Value"=w206:T10)  [unwired: 2 in, 2 out]
        n145 = property on="Color Space" class="Enum （指定）"() -> ("Value"=w208:T9)  [unwired: 2 in, 2 out]
        n146 = property on="Type of Calibration" class="RadioBtnsControl （指定）"() -> ("Value"=w204:enum32{"Single-Point", "RGB", "WRGB"})  [unwired: 2 in, 2 out]
        n147 = Add(x=w206, y=1) -> (x+y=w205:i32)
        n148 = case shown="\"Lv,u',v'\"" w208 {
          selector: w208 -> [w217 w369 w518 w667 w816]
          tunnel: w207 -> [w224 w376 w525 w674 w823]
          tunnel: w205 -> [w223 w375 w524 w673 w822]
          tunnel: "ID" -> [w222 w374 w523 w672 w821]
          tunnel: w204 -> [w213 w367 w516 w665 w814]
          tunnel: "タイムスタンプ" -> [w214 w368 w517 w666 w815]
          frame "Lv,u',v'" {
            n149 = case shown="\"WRGB\"" w213 {
              tunnel: w217 -> [w235 w265 w319]
              tunnel: [w234 w255 w312] -> w216
              tunnel: [w232 w250 w309] -> w215
              tunnel: w214 -> [w228 w263 w317]
              frame "Single-Point", Default {
                n150 = flat-sequence {
                  tunnel: w235 -> [w244]
                  tunnel: [w240] -> w233
                  tunnel: [w239] -> w231
                  tunnel: [w238] -> w230
                  tunnel: [w237] -> w229
                  tunnel: w228 -> [w236]
                  frame #0 {
                    n151 = property on="After_W" class="Clust （指定）"() -> ("Value"=w248:T4)  [unwired: 2 in, 2 out]
                    n152 = Unbundle(w248) -> ("After_W1"=w243:dbl, "After_W2"=w242:dbl, "After_W3"=w241:dbl)
                    n153 = property on="Before_W" class="Clust （指定）"() -> ("Value"=w249:T8)  [unwired: 2 in, 2 out]
                    n154 = Unbundle(w249) -> ("before_W1"=w247:dbl, "Before_W2"=w246:dbl, "Before_W3"=w245:dbl)
                    n155 = call "LC-MISDK_UserCalibration_MakeListData_Lvuv.vi"("Before_2"=w242, "Before_3"=w241, "before_1"=w243, "タイムスタンプ"=w236, "Value"=w244) -> ("リファレンス出力"=w239:refnum<k24>, ".NET refnum出力"=w240:refnum<k24>)  [unwired: 5 in]
                    n156 = call "LC-MISDK_UserCalibration_MakeListData_Lvuv.vi"("Before_2"=w246, "Before_3"=w245, "before_1"=w247, "タイムスタンプ"=w236, "Value"=w244) -> ("リファレンス出力"=w237:refnum<k24>, ".NET refnum出力"=w238:refnum<k24>)  [unwired: 5 in]
                  }
                }
                n157 = invoke on="インボークノード" class="List`1[[Konicaminolta.Lvudvd, L" method="Add"(reference=w229, "item"=w230) -> (reference out=w234:refnum<k24>)  [unwired: 2 in, 3 out]
                n158 = invoke on="インボークノード" class="List`1[[Konicaminolta.Lvudvd, L" method="Add"(reference=w231, "item"=w233) -> (reference out=w232:refnum<k24>)  [unwired: 2 in, 3 out]
              }
              frame "RGB" {
                n159 = flat-sequence {
                  tunnel: w265 -> [w271]
                  tunnel: [w293] -> w264
                  tunnel: [w292] -> w260
                  tunnel: w263 -> [w273]
                  tunnel: [w276] -> w262
                  tunnel: [w275] -> w261
                  tunnel: [w269] -> w259
                  tunnel: [w268] -> w257
                  tunnel: [w267] -> w253
                  tunnel: [w266] -> w251
                  frame #0 {
                    n160 = property on="After_R" class="Clust （指定）"() -> ("Value"=w290:T3)  [unwired: 2 in, 2 out]
                    n161 = property on="After_B" class="Clust （指定）"() -> ("Value"=w274:T1)  [unwired: 2 in, 2 out]
                    n162 = property on="After_G" class="Clust （指定）"() -> ("Value"=w270:T2)  [unwired: 2 in, 2 out]
                    n163 = property on="Before_R" class="Clust （指定）"() -> ("Value"=w291:T7)  [unwired: 2 in, 2 out]
                    n164 = property on="Before_G" class="Clust （指定）"() -> ("Value"=w286:T6)  [unwired: 2 in, 2 out]
                    n165 = property on="Before_B" class="Clust （指定）"() -> ("Value"=w282:T5)  [unwired: 2 in, 2 out]
                    n166 = Unbundle(w290) -> ("After_R1"=w296:dbl, "After_R2"=w295:dbl, "After_R3"=w294:dbl)
                    n167 = Unbundle(w270) -> ("After_G1"=w281:dbl, "After_G2"=w280:dbl, "After_G3"=w279:dbl)
                    n168 = Unbundle(w274) -> ("After_B1"=w278:dbl, "After_B2"=w277:dbl, "After_B3"=w272:dbl)
                    n169 = Unbundle(w291) -> ("before_R1"=w299:dbl, "Before_R2"=w298:dbl, "Before_R3"=w297:dbl)
                    n170 = Unbundle(w286) -> ("before_G1"=w289:dbl, "Before_G2"=w288:dbl, "Before_G3"=w287:dbl)
                    n171 = Unbundle(w282) -> ("before_B1"=w285:dbl, "Before_B2"=w284:dbl, "Before_B3"=w283:dbl)
                    n172 = call "LC-MISDK_UserCalibration_MakeListData_Lvuv.vi"("Before_2"=w298, "Before_3"=w297, "before_1"=w299, "タイムスタンプ"=w273, "Value"=w271) -> ("リファレンス出力"=w292:refnum<k24>, ".NET refnum出力"=w293:refnum<k24>)  [unwired: 5 in]
                    n173 = call "LC-MISDK_UserCalibration_MakeListData_Lvuv.vi"("Before_2"=w288, "Before_3"=w287, "before_1"=w289, "タイムスタンプ"=w273, "Value"=w271) -> (".NET refnum出力"=w269:refnum<k24>)  [unwired: 5 in, 1 out]
                    n174 = call "LC-MISDK_UserCalibration_MakeListData_Lvuv.vi"("Before_2"=w295, "Before_3"=w294, "before_1"=w296, "タイムスタンプ"=w273, "Value"=w271) -> ("リファレンス出力"=w275:refnum<k24>, ".NET refnum出力"=w276:refnum<k24>)  [unwired: 5 in]
                    n175 = call "LC-MISDK_UserCalibration_MakeListData_Lvuv.vi"("Before_2"=w284, "Before_3"=w283, "before_1"=w285, "タイムスタンプ"=w273, "Value"=w271) -> (".NET refnum出力"=w268:refnum<k24>)  [unwired: 5 in, 1 out]
                    n176 = call "LC-MISDK_UserCalibration_MakeListData_Lvuv.vi"("Before_2"=w280, "Before_3"=w279, "before_1"=w281, "タイムスタンプ"=w273, "Value"=w271) -> (".NET refnum出力"=w267:refnum<k24>)  [unwired: 5 in, 1 out]
                    n177 = call "LC-MISDK_UserCalibration_MakeListData_Lvuv.vi"("Before_2"=w277, "Before_3"=w272, "before_1"=w278, "タイムスタンプ"=w273, "Value"=w271) -> (".NET refnum出力"=w266:refnum<k24>)  [unwired: 5 in, 1 out]
                  }
                }
                n178 = invoke on="インボークノード" class="List`1[[Konicaminolta.Lvudvd, L" method="Add"(reference=w260, "item"=w264) -> (reference out=w258:refnum<k24>)  [unwired: 2 in, 3 out]
                n179 = invoke on="インボークノード" class="List`1[[Konicaminolta.Lvudvd, L" method="Add"(reference=w258, "item"=w259) -> (reference out=w256:refnum<k24>)  [unwired: 2 in, 3 out]
                n180 = invoke on="インボークノード" class="List`1[[Konicaminolta.Lvudvd, L" method="Add"(reference=w256, "item"=w257) -> (reference out=w255:refnum<k24>)  [unwired: 2 in, 3 out]
                n181 = invoke on="インボークノード" class="List`1[[Konicaminolta.Lvudvd, L" method="Add"(reference=w261, "item"=w262) -> (reference out=w254:refnum<k24>)  [unwired: 2 in, 3 out]
                n182 = invoke on="インボークノード" class="List`1[[Konicaminolta.Lvudvd, L" method="Add"(reference=w254, "item"=w253) -> (reference out=w252:refnum<k24>)  [unwired: 2 in, 3 out]
                n183 = invoke on="インボークノード" class="List`1[[Konicaminolta.Lvudvd, L" method="Add"(reference=w252, "item"=w251) -> (reference out=w250:refnum<k24>)  [unwired: 2 in, 3 out]
              }
              frame "WRGB" {
                n184 = flat-sequence {
                  tunnel: w319 -> [w328]
                  tunnel: [w357] -> w318
                  tunnel: w317 -> [w327]
                  tunnel: [w338] -> w316
                  tunnel: [w337] -> w314
                  tunnel: [w326] -> w307
                  tunnel: [w325] -> w306
                  tunnel: [w324] -> w305
                  tunnel: [w323] -> w304
                  tunnel: [w322] -> w302
                  tunnel: [w321] -> w301
                  tunnel: [w320] -> w300
                  frame #0 {
                    n185 = property on="After_R" class="Clust （指定）"() -> ("Value"=w355:T3)  [unwired: 2 in, 2 out]
                    n186 = property on="After_B" class="Clust （指定）"() -> ("Value"=w341:T1)  [unwired: 2 in, 2 out]
                    n187 = property on="After_G" class="Clust （指定）"() -> ("Value"=w339:T2)  [unwired: 2 in, 2 out]
                    n188 = property on="Before_W" class="Clust （指定）"() -> ("Value"=w333:T8)  [unwired: 2 in, 2 out]
                    n189 = property on="Before_R" class="Clust （指定）"() -> ("Value"=w356:T7)  [unwired: 2 in, 2 out]
                    n190 = property on="Before_G" class="Clust （指定）"() -> ("Value"=w351:T6)  [unwired: 2 in, 2 out]
                    n191 = property on="Before_B" class="Clust （指定）"() -> ("Value"=w347:T5)  [unwired: 2 in, 2 out]
                    n192 = property on="After_W" class="Clust （指定）"() -> ("Value"=w329:T4)  [unwired: 2 in, 2 out]
                    n193 = Unbundle(w355) -> ("After_R1"=w360:dbl, "After_R2"=w359:dbl, "After_R3"=w358:dbl)
                    n194 = Unbundle(w339) -> ("After_G1"=w346:dbl, "After_G2"=w345:dbl, "After_G3"=w344:dbl)
                    n195 = Unbundle(w341) -> ("After_B1"=w343:dbl, "After_B2"=w342:dbl, "After_B3"=w340:dbl)
                    n196 = Unbundle(w333) -> ("before_W1"=w336:dbl, "Before_W2"=w335:dbl, "Before_W3"=w334:dbl)
                    n197 = Unbundle(w356) -> ("before_R1"=w363:dbl, "Before_R2"=w362:dbl, "Before_R3"=w361:dbl)
                    n198 = Unbundle(w351) -> ("before_G1"=w354:dbl, "Before_G2"=w353:dbl, "Before_G3"=w352:dbl)
                    n199 = Unbundle(w329) -> ("After_W1"=w330:dbl, "After_W2"=w331:dbl, "After_W3"=w332:dbl)
                    n200 = Unbundle(w347) -> ("before_B1"=w350:dbl, "Before_B2"=w349:dbl, "Before_B3"=w348:dbl)
                    n201 = call "LC-MISDK_UserCalibration_MakeListData_Lvuv.vi"("Before_2"=w335, "Before_3"=w334, "before_1"=w336, "タイムスタンプ"=w327, "Value"=w328) -> ("リファレンス出力"=w325:refnum<k24>, ".NET refnum出力"=w326:refnum<k24>)  [unwired: 5 in]
                    n202 = call "LC-MISDK_UserCalibration_MakeListData_Lvuv.vi"("Before_2"=w362, "Before_3"=w361, "before_1"=w363, "タイムスタンプ"=w327, "Value"=w328) -> (".NET refnum出力"=w357:refnum<k24>)  [unwired: 5 in, 1 out]
                    n203 = call "LC-MISDK_UserCalibration_MakeListData_Lvuv.vi"("Before_2"=w353, "Before_3"=w352, "before_1"=w354, "タイムスタンプ"=w327, "Value"=w328) -> (".NET refnum出力"=w338:refnum<k24>)  [unwired: 5 in, 1 out]
                    n204 = call "LC-MISDK_UserCalibration_MakeListData_Lvuv.vi"("Before_2"=w359, "Before_3"=w358, "before_1"=w360, "タイムスタンプ"=w327, "Value"=w328) -> (".NET refnum出力"=w322:refnum<k24>)  [unwired: 5 in, 1 out]
                    n205 = call "LC-MISDK_UserCalibration_MakeListData_Lvuv.vi"("Before_2"=w331, "Before_3"=w332, "before_1"=w330, "タイムスタンプ"=w327, "Value"=w328) -> ("リファレンス出力"=w323:refnum<k24>, ".NET refnum出力"=w324:refnum<k24>)  [unwired: 5 in]
                    n206 = call "LC-MISDK_UserCalibration_MakeListData_Lvuv.vi"("Before_2"=w349, "Before_3"=w348, "before_1"=w350, "タイムスタンプ"=w327, "Value"=w328) -> (".NET refnum出力"=w337:refnum<k24>)  [unwired: 5 in, 1 out]
                    n207 = call "LC-MISDK_UserCalibration_MakeListData_Lvuv.vi"("Before_2"=w345, "Before_3"=w344, "before_1"=w346, "タイムスタンプ"=w327, "Value"=w328) -> (".NET refnum出力"=w321:refnum<k24>)  [unwired: 5 in, 1 out]
                    n208 = call "LC-MISDK_UserCalibration_MakeListData_Lvuv.vi"("Before_2"=w342, "Before_3"=w340, "before_1"=w343, "タイムスタンプ"=w327, "Value"=w328) -> (".NET refnum出力"=w320:refnum<k24>)  [unwired: 5 in, 1 out]
                  }
                }
                n209 = invoke on="インボークノード" class="List`1[[Konicaminolta.Lvudvd, L" method="Add"(reference=w304, "item"=w305) -> (reference out=w303:refnum<k24>)  [unwired: 2 in, 3 out]
                n210 = invoke on="インボークノード" class="List`1[[Konicaminolta.Lvudvd, L" method="Add"(reference=w306, "item"=w307) -> (reference out=w308:refnum<k24>)  [unwired: 2 in, 3 out]
                n211 = invoke on="インボークノード" class="List`1[[Konicaminolta.Lvudvd, L" method="Add"(reference=w308, "item"=w318) -> (reference out=w315:refnum<k24>)  [unwired: 2 in, 3 out]
                n212 = invoke on="インボークノード" class="List`1[[Konicaminolta.Lvudvd, L" method="Add"(reference=w315, "item"=w316) -> (reference out=w313:refnum<k24>)  [unwired: 2 in, 3 out]
                n213 = invoke on="インボークノード" class="List`1[[Konicaminolta.Lvudvd, L" method="Add"(reference=w313, "item"=w314) -> (reference out=w312:refnum<k24>)  [unwired: 2 in, 3 out]
                n214 = invoke on="インボークノード" class="List`1[[Konicaminolta.Lvudvd, L" method="Add"(reference=w303, "item"=w302) -> (reference out=w311:refnum<k24>)  [unwired: 2 in, 3 out]
                n215 = invoke on="インボークノード" class="List`1[[Konicaminolta.Lvudvd, L" method="Add"(reference=w311, "item"=w301) -> (reference out=w310:refnum<k24>)  [unwired: 2 in, 3 out]
                n216 = invoke on="インボークノード" class="List`1[[Konicaminolta.Lvudvd, L" method="Add"(reference=w310, "item"=w300) -> (reference out=w309:refnum<k24>)  [unwired: 2 in, 3 out]
              }
            }
            n217 = invoke on="インボークノード" class="LightColorMISDK" method="SetMatrixCalib"(reference=w224, "calibrationCh"=w223, "measurementDataList"=w216, "correctDataList"=w215, "type"=w213, "id"=w222, "comPort"=0) -> (error out=w220:errorcluster, "SetMatrixCalib"=w221:refnum<k24>)  [unwired: 2 in, 7 out]
            n218 = property on="プロパティノード" class="ReturnMessage"(reference=w221, error in=w220) -> (reference out=w210:refnum<k24>, error out=w219:errorcluster, "errorCode"=w211:i32)
            "CalError" <- w211
            n219 = Not Equal To 0?(x=w211) -> (x != 0?=w212:bool)
            n220 = property on="error out" class="Clust （指定）"("Value"=w219) -> ()  [unwired: 2 in, 2 out]
            n221 = case shown="TRUE" w212 {
              tunnel: w210 -> [_ w225]
              frame False {
              }
              frame True {
                n222 = property on="プロパティノード" class="ReturnMessage"(reference=w225) -> (error out=w227:errorcluster, "errorMessage"=w226:refnum<k24>)  [unwired: 1 in, 1 out]
                n223 = invoke class="List`1[[System.String, mscorlib" method="ToString"(reference=w226, error in=w227) -> ()  [unwired: 1 in, 3 out]
              }
            }
          }
          frame "Lv,Tcp,duv" {
            n224 = case shown="\"WRGB\"" w367 {
              tunnel: w369 -> [w384 w414 w468]
              tunnel: [w383 w400 w450] -> w366
              tunnel: [w381 w399 w449] -> w365
              tunnel: w368 -> [w377 w412 w466]
              frame "Single-Point", Default {
                n225 = flat-sequence {
                  tunnel: w384 -> [w393]
                  tunnel: [w389] -> w382
                  tunnel: [w388] -> w380
                  tunnel: [w387] -> w379
                  tunnel: [w386] -> w378
                  tunnel: w377 -> [w385]
                  frame #0 {
                    n226 = property on="After_W" class="Clust （指定）"() -> ("Value"=w397:T4)  [unwired: 2 in, 2 out]
                    n227 = Unbundle(w397) -> ("After_W1"=w392:dbl, "After_W2"=w391:dbl, "After_W3"=w390:dbl)
                    n228 = property on="Before_W" class="Clust （指定）"() -> ("Value"=w398:T8)  [unwired: 2 in, 2 out]
                    n229 = Unbundle(w398) -> ("before_W1"=w396:dbl, "Before_W2"=w395:dbl, "Before_W3"=w394:dbl)
                    n230 = call "LC-MISDK_UserCalibration_MakeListData_LvTcpduv.vi"("Before_2"=w391, "Before_3"=w390, "before_1"=w392, "タイムスタンプ"=w385, "Value"=w393) -> ("リファレンス出力"=w388:refnum<k24>, ".NET refnum出力"=w389:refnum<k24>)  [unwired: 5 in]
                    n231 = call "LC-MISDK_UserCalibration_MakeListData_LvTcpduv.vi"("Before_2"=w395, "Before_3"=w394, "before_1"=w396, "タイムスタンプ"=w385, "Value"=w393) -> ("リファレンス出力"=w386:refnum<k24>, ".NET refnum出力"=w387:refnum<k24>)  [unwired: 5 in]
                  }
                }
                n232 = invoke on="インボークノード" class="List`1[[Konicaminolta.LvTcpDuv," method="Add"(reference=w378, "item"=w379) -> (reference out=w383:refnum<k24>)  [unwired: 2 in, 3 out]
                n233 = invoke on="インボークノード" class="List`1[[Konicaminolta.LvTcpDuv," method="Add"(reference=w380, "item"=w382) -> (reference out=w381:refnum<k24>)  [unwired: 2 in, 3 out]
              }
              frame "RGB" {
                n234 = flat-sequence {
                  tunnel: w414 -> [w420]
                  tunnel: [w442] -> w413
                  tunnel: [w441] -> w409
                  tunnel: w412 -> [w422]
                  tunnel: [w425] -> w411
                  tunnel: [w424] -> w410
                  tunnel: [w418] -> w408
                  tunnel: [w417] -> w406
                  tunnel: [w416] -> w403
                  tunnel: [w415] -> w401
                  frame #0 {
                    n235 = property on="After_R" class="Clust （指定）"() -> ("Value"=w439:T3)  [unwired: 2 in, 2 out]
                    n236 = property on="After_B" class="Clust （指定）"() -> ("Value"=w423:T1)  [unwired: 2 in, 2 out]
                    n237 = property on="After_G" class="Clust （指定）"() -> ("Value"=w419:T2)  [unwired: 2 in, 2 out]
                    n238 = property on="Before_R" class="Clust （指定）"() -> ("Value"=w440:T7)  [unwired: 2 in, 2 out]
                    n239 = property on="Before_G" class="Clust （指定）"() -> ("Value"=w435:T6)  [unwired: 2 in, 2 out]
                    n240 = property on="Before_B" class="Clust （指定）"() -> ("Value"=w431:T5)  [unwired: 2 in, 2 out]
                    n241 = Unbundle(w439) -> ("After_R1"=w445:dbl, "After_R2"=w444:dbl, "After_R3"=w443:dbl)
                    n242 = Unbundle(w419) -> ("After_G1"=w430:dbl, "After_G2"=w429:dbl, "After_G3"=w428:dbl)
                    n243 = Unbundle(w423) -> ("After_B1"=w427:dbl, "After_B2"=w426:dbl, "After_B3"=w421:dbl)
                    n244 = Unbundle(w440) -> ("before_R1"=w448:dbl, "Before_R2"=w447:dbl, "Before_R3"=w446:dbl)
                    n245 = Unbundle(w435) -> ("before_G1"=w438:dbl, "Before_G2"=w437:dbl, "Before_G3"=w436:dbl)
                    n246 = Unbundle(w431) -> ("before_B1"=w434:dbl, "Before_B2"=w433:dbl, "Before_B3"=w432:dbl)
                    n247 = call "LC-MISDK_UserCalibration_MakeListData_LvTcpduv.vi"("Before_2"=w447, "Before_3"=w446, "before_1"=w448, "タイムスタンプ"=w422, "Value"=w420) -> ("リファレンス出力"=w441:refnum<k24>, ".NET refnum出力"=w442:refnum<k24>)  [unwired: 5 in]
                    n248 = call "LC-MISDK_UserCalibration_MakeListData_LvTcpduv.vi"("Before_2"=w437, "Before_3"=w436, "before_1"=w438, "タイムスタンプ"=w422, "Value"=w420) -> (".NET refnum出力"=w418:refnum<k24>)  [unwired: 5 in, 1 out]
                    n249 = call "LC-MISDK_UserCalibration_MakeListData_LvTcpduv.vi"("Before_2"=w444, "Before_3"=w443, "before_1"=w445, "タイムスタンプ"=w422, "Value"=w420) -> ("リファレンス出力"=w424:refnum<k24>, ".NET refnum出力"=w425:refnum<k24>)  [unwired: 5 in]
                    n250 = call "LC-MISDK_UserCalibration_MakeListData_LvTcpduv.vi"("Before_2"=w433, "Before_3"=w432, "before_1"=w434, "タイムスタンプ"=w422, "Value"=w420) -> (".NET refnum出力"=w417:refnum<k24>)  [unwired: 5 in, 1 out]
                    n251 = call "LC-MISDK_UserCalibration_MakeListData_LvTcpduv.vi"("Before_2"=w429, "Before_3"=w428, "before_1"=w430, "タイムスタンプ"=w422, "Value"=w420) -> (".NET refnum出力"=w416:refnum<k24>)  [unwired: 5 in, 1 out]
                    n252 = call "LC-MISDK_UserCalibration_MakeListData_LvTcpduv.vi"("Before_2"=w426, "Before_3"=w421, "before_1"=w427, "タイムスタンプ"=w422, "Value"=w420) -> (".NET refnum出力"=w415:refnum<k24>)  [unwired: 5 in, 1 out]
                  }
                }
                n253 = invoke on="インボークノード" class="List`1[[Konicaminolta.LvTcpDuv," method="Add"(reference=w409, "item"=w413) -> (reference out=w407:refnum<k24>)  [unwired: 2 in, 3 out]
                n254 = invoke on="インボークノード" class="List`1[[Konicaminolta.LvTcpDuv," method="Add"(reference=w407, "item"=w408) -> (reference out=w405:refnum<k24>)  [unwired: 2 in, 3 out]
                n255 = invoke on="インボークノード" class="List`1[[Konicaminolta.LvTcpDuv," method="Add"(reference=w405, "item"=w406) -> (reference out=w400:refnum<k24>)  [unwired: 2 in, 3 out]
                n256 = invoke on="インボークノード" class="List`1[[Konicaminolta.LvTcpDuv," method="Add"(reference=w410, "item"=w411) -> (reference out=w404:refnum<k24>)  [unwired: 2 in, 3 out]
                n257 = invoke on="インボークノード" class="List`1[[Konicaminolta.LvTcpDuv," method="Add"(reference=w404, "item"=w403) -> (reference out=w402:refnum<k24>)  [unwired: 2 in, 3 out]
                n258 = invoke on="インボークノード" class="List`1[[Konicaminolta.LvTcpDuv," method="Add"(reference=w402, "item"=w401) -> (reference out=w399:refnum<k24>)  [unwired: 2 in, 3 out]
              }
              frame "WRGB" {
                n259 = flat-sequence {
                  tunnel: w468 -> [w471]
                  tunnel: [w506] -> w467
                  tunnel: w466 -> [w474]
                  tunnel: [w487] -> w465
                  tunnel: [w486] -> w463
                  tunnel: [w480] -> w458
                  tunnel: [w479] -> w457
                  tunnel: [w478] -> w455
                  tunnel: [w477] -> w454
                  tunnel: [w476] -> w453
                  tunnel: [w470] -> w452
                  tunnel: [w469] -> w451
                  frame #0 {
                    n260 = property on="After_R" class="Clust （指定）"() -> ("Value"=w504:T3)  [unwired: 2 in, 2 out]
                    n261 = property on="After_B" class="Clust （指定）"() -> ("Value"=w490:T1)  [unwired: 2 in, 2 out]
                    n262 = property on="After_G" class="Clust （指定）"() -> ("Value"=w488:T2)  [unwired: 2 in, 2 out]
                    n263 = property on="Before_W" class="Clust （指定）"() -> ("Value"=w485:T8)  [unwired: 2 in, 2 out]
                    n264 = property on="Before_R" class="Clust （指定）"() -> ("Value"=w505:T7)  [unwired: 2 in, 2 out]
                    n265 = property on="Before_G" class="Clust （指定）"() -> ("Value"=w500:T6)  [unwired: 2 in, 2 out]
                    n266 = property on="Before_B" class="Clust （指定）"() -> ("Value"=w496:T5)  [unwired: 2 in, 2 out]
                    n267 = property on="After_W" class="Clust （指定）"() -> ("Value"=w481:T4)  [unwired: 2 in, 2 out]
                    n268 = Unbundle(w504) -> ("After_R1"=w509:dbl, "After_R2"=w508:dbl, "After_R3"=w507:dbl)
                    n269 = Unbundle(w488) -> ("After_G1"=w495:dbl, "After_G2"=w494:dbl, "After_G3"=w493:dbl)
                    n270 = Unbundle(w490) -> ("After_B1"=w492:dbl, "After_B2"=w491:dbl, "After_B3"=w489:dbl)
                    n271 = Unbundle(w485) -> ("before_W1"=w473:dbl, "Before_W2"=w475:dbl, "Before_W3"=w472:dbl)
                    n272 = Unbundle(w505) -> ("before_R1"=w512:dbl, "Before_R2"=w511:dbl, "Before_R3"=w510:dbl)
                    n273 = Unbundle(w500) -> ("before_G1"=w503:dbl, "Before_G2"=w502:dbl, "Before_G3"=w501:dbl)
                    n274 = Unbundle(w481) -> ("After_W1"=w482:dbl, "After_W2"=w483:dbl, "After_W3"=w484:dbl)
                    n275 = Unbundle(w496) -> ("before_B1"=w499:dbl, "Before_B2"=w498:dbl, "Before_B3"=w497:dbl)
                    n276 = call "LC-MISDK_UserCalibration_MakeListData_LvTcpduv.vi"("Before_2"=w511, "Before_3"=w510, "before_1"=w512, "タイムスタンプ"=w474, "Value"=w471) -> (".NET refnum出力"=w506:refnum<k24>)  [unwired: 5 in, 1 out]
                    n277 = call "LC-MISDK_UserCalibration_MakeListData_LvTcpduv.vi"("Before_2"=w475, "Before_3"=w472, "before_1"=w473, "タイムスタンプ"=w474, "Value"=w471) -> ("リファレンス出力"=w469:refnum<k24>, ".NET refnum出力"=w470:refnum<k24>)  [unwired: 5 in]
                    n278 = call "LC-MISDK_UserCalibration_MakeListData_LvTcpduv.vi"("Before_2"=w502, "Before_3"=w501, "before_1"=w503, "タイムスタンプ"=w474, "Value"=w471) -> (".NET refnum出力"=w487:refnum<k24>)  [unwired: 5 in, 1 out]
                    n279 = call "LC-MISDK_UserCalibration_MakeListData_LvTcpduv.vi"("Before_2"=w508, "Before_3"=w507, "before_1"=w509, "タイムスタンプ"=w474, "Value"=w471) -> (".NET refnum出力"=w478:refnum<k24>)  [unwired: 5 in, 1 out]
                    n280 = call "LC-MISDK_UserCalibration_MakeListData_LvTcpduv.vi"("Before_2"=w483, "Before_3"=w484, "before_1"=w482, "タイムスタンプ"=w474, "Value"=w471) -> ("リファレンス出力"=w479:refnum<k24>, ".NET refnum出力"=w480:refnum<k24>)  [unwired: 5 in]
                    n281 = call "LC-MISDK_UserCalibration_MakeListData_LvTcpduv.vi"("Before_2"=w498, "Before_3"=w497, "before_1"=w499, "タイムスタンプ"=w474, "Value"=w471) -> (".NET refnum出力"=w486:refnum<k24>)  [unwired: 5 in, 1 out]
                    n282 = call "LC-MISDK_UserCalibration_MakeListData_LvTcpduv.vi"("Before_2"=w494, "Before_3"=w493, "before_1"=w495, "タイムスタンプ"=w474, "Value"=w471) -> (".NET refnum出力"=w477:refnum<k24>)  [unwired: 5 in, 1 out]
                    n283 = call "LC-MISDK_UserCalibration_MakeListData_LvTcpduv.vi"("Before_2"=w491, "Before_3"=w489, "before_1"=w492, "タイムスタンプ"=w474, "Value"=w471) -> (".NET refnum出力"=w476:refnum<k24>)  [unwired: 5 in, 1 out]
                  }
                }
                n284 = invoke on="インボークノード" class="List`1[[Konicaminolta.LvTcpDuv," method="Add"(reference=w457, "item"=w458) -> (reference out=w456:refnum<k24>)  [unwired: 2 in, 3 out]
                n285 = invoke on="インボークノード" class="List`1[[Konicaminolta.LvTcpDuv," method="Add"(reference=w451, "item"=w452) -> (reference out=w459:refnum<k24>)  [unwired: 2 in, 3 out]
                n286 = invoke on="インボークノード" class="List`1[[Konicaminolta.LvTcpDuv," method="Add"(reference=w459, "item"=w467) -> (reference out=w464:refnum<k24>)  [unwired: 2 in, 3 out]
                n287 = invoke on="インボークノード" class="List`1[[Konicaminolta.LvTcpDuv," method="Add"(reference=w464, "item"=w465) -> (reference out=w462:refnum<k24>)  [unwired: 2 in, 3 out]
                n288 = invoke on="インボークノード" class="List`1[[Konicaminolta.LvTcpDuv," method="Add"(reference=w462, "item"=w463) -> (reference out=w450:refnum<k24>)  [unwired: 2 in, 3 out]
                n289 = invoke on="インボークノード" class="List`1[[Konicaminolta.LvTcpDuv," method="Add"(reference=w456, "item"=w455) -> (reference out=w461:refnum<k24>)  [unwired: 2 in, 3 out]
                n290 = invoke on="インボークノード" class="List`1[[Konicaminolta.LvTcpDuv," method="Add"(reference=w461, "item"=w454) -> (reference out=w460:refnum<k24>)  [unwired: 2 in, 3 out]
                n291 = invoke on="インボークノード" class="List`1[[Konicaminolta.LvTcpDuv," method="Add"(reference=w460, "item"=w453) -> (reference out=w449:refnum<k24>)  [unwired: 2 in, 3 out]
              }
            }
            n292 = invoke on="インボークノード" class="LightColorMISDK" method="SetMatrixCalib"(reference=w376, "calibrationCh"=w375, "measurementDataList"=w366, "correctDataList"=w365, "type"=w367, "id"=w374, "comPort"=0) -> (error out=w372:errorcluster, "SetMatrixCalib"=w373:refnum<k24>)  [unwired: 2 in, 7 out]
            n293 = property on="プロパティノード" class="ReturnMessage"(reference=w373, error in=w372) -> (error out=w371:errorcluster, "errorCode"=w364:i32)  [unwired: 1 out]
            n294 = property on="error out" class="Clust （指定）"("Value"=w371) -> ()  [unwired: 2 in, 2 out]
            n295 = property on="CalError" class="DigNum （指定）"("Value"=w364) -> ()  [unwired: 2 in, 2 out]
          }
          frame "X,Y,Z" {
            n296 = case shown="\"Single-Point\", デフォルト" w516 {
              tunnel: w518 -> [w533 w563 w617]
              tunnel: [w532 w549 w599] -> w515
              tunnel: [w530 w548 w598] -> w514
              tunnel: w517 -> [w526 w561 w615]
              frame "Single-Point", Default {
                n297 = flat-sequence {
                  tunnel: w533 -> [w542]
                  tunnel: [w538] -> w531
                  tunnel: [w537] -> w529
                  tunnel: [w536] -> w528
                  tunnel: [w535] -> w527
                  tunnel: w526 -> [w534]
                  frame #0 {
                    n298 = property on="After_W" class="Clust （指定）"() -> ("Value"=w546:T4)  [unwired: 2 in, 2 out]
                    n299 = Unbundle(w546) -> ("After_W1"=w541:dbl, "After_W2"=w540:dbl, "After_W3"=w539:dbl)
                    n300 = property on="Before_W" class="Clust （指定）"() -> ("Value"=w547:T8)  [unwired: 2 in, 2 out]
                    n301 = Unbundle(w547) -> ("before_W1"=w545:dbl, "Before_W2"=w544:dbl, "Before_W3"=w543:dbl)
                    n302 = call "LC-MISDK_UserCalibration_MakeListData_XYZ.vi"("Before_2"=w540, "Before_3"=w539, "before_1"=w541, "タイムスタンプ"=w534, "Value"=w542) -> ("リファレンス出力"=w537:refnum<k24>, ".NET refnum出力"=w538:refnum<k24>)  [unwired: 5 in]
                    n303 = call "LC-MISDK_UserCalibration_MakeListData_XYZ.vi"("Before_2"=w544, "Before_3"=w543, "before_1"=w545, "タイムスタンプ"=w534, "Value"=w542) -> ("リファレンス出力"=w535:refnum<k24>, ".NET refnum出力"=w536:refnum<k24>)  [unwired: 5 in]
                  }
                }
                n304 = invoke on="インボークノード" class="List`1[[Konicaminolta.XYZ, LC-M" method="Add"(reference=w527, "item"=w528) -> (reference out=w532:refnum<k24>)  [unwired: 2 in, 3 out]
                n305 = invoke on="インボークノード" class="List`1[[Konicaminolta.XYZ, LC-M" method="Add"(reference=w529, "item"=w531) -> (reference out=w530:refnum<k24>)  [unwired: 2 in, 3 out]
              }
              frame "RGB" {
                n306 = flat-sequence {
                  tunnel: w563 -> [w569]
                  tunnel: [w591] -> w562
                  tunnel: [w590] -> w558
                  tunnel: w561 -> [w571]
                  tunnel: [w574] -> w560
                  tunnel: [w573] -> w559
                  tunnel: [w567] -> w557
                  tunnel: [w566] -> w555
                  tunnel: [w565] -> w552
                  tunnel: [w564] -> w550
                  frame #0 {
                    n307 = property on="After_R" class="Clust （指定）"() -> ("Value"=w588:T3)  [unwired: 2 in, 2 out]
                    n308 = property on="After_B" class="Clust （指定）"() -> ("Value"=w572:T1)  [unwired: 2 in, 2 out]
                    n309 = property on="After_G" class="Clust （指定）"() -> ("Value"=w568:T2)  [unwired: 2 in, 2 out]
                    n310 = property on="Before_R" class="Clust （指定）"() -> ("Value"=w589:T7)  [unwired: 2 in, 2 out]
                    n311 = property on="Before_G" class="Clust （指定）"() -> ("Value"=w584:T6)  [unwired: 2 in, 2 out]
                    n312 = property on="Before_B" class="Clust （指定）"() -> ("Value"=w580:T5)  [unwired: 2 in, 2 out]
                    n313 = Unbundle(w588) -> ("After_R1"=w594:dbl, "After_R2"=w593:dbl, "After_R3"=w592:dbl)
                    n314 = Unbundle(w568) -> ("After_G1"=w579:dbl, "After_G2"=w578:dbl, "After_G3"=w577:dbl)
                    n315 = Unbundle(w572) -> ("After_B1"=w576:dbl, "After_B2"=w575:dbl, "After_B3"=w570:dbl)
                    n316 = Unbundle(w589) -> ("before_R1"=w597:dbl, "Before_R2"=w596:dbl, "Before_R3"=w595:dbl)
                    n317 = Unbundle(w584) -> ("before_G1"=w587:dbl, "Before_G2"=w586:dbl, "Before_G3"=w585:dbl)
                    n318 = Unbundle(w580) -> ("before_B1"=w583:dbl, "Before_B2"=w582:dbl, "Before_B3"=w581:dbl)
                    n319 = call "LC-MISDK_UserCalibration_MakeListData_XYZ.vi"("Before_2"=w596, "Before_3"=w595, "before_1"=w597, "タイムスタンプ"=w571, "Value"=w569) -> ("リファレンス出力"=w590:refnum<k24>, ".NET refnum出力"=w591:refnum<k24>)  [unwired: 5 in]
                    n320 = call "LC-MISDK_UserCalibration_MakeListData_XYZ.vi"("Before_2"=w586, "Before_3"=w585, "before_1"=w587, "タイムスタンプ"=w571, "Value"=w569) -> (".NET refnum出力"=w567:refnum<k24>)  [unwired: 5 in, 1 out]
                    n321 = call "LC-MISDK_UserCalibration_MakeListData_XYZ.vi"("Before_2"=w593, "Before_3"=w592, "before_1"=w594, "タイムスタンプ"=w571, "Value"=w569) -> ("リファレンス出力"=w573:refnum<k24>, ".NET refnum出力"=w574:refnum<k24>)  [unwired: 5 in]
                    n322 = call "LC-MISDK_UserCalibration_MakeListData_XYZ.vi"("Before_2"=w582, "Before_3"=w581, "before_1"=w583, "タイムスタンプ"=w571, "Value"=w569) -> (".NET refnum出力"=w566:refnum<k24>)  [unwired: 5 in, 1 out]
                    n323 = call "LC-MISDK_UserCalibration_MakeListData_XYZ.vi"("Before_2"=w578, "Before_3"=w577, "before_1"=w579, "タイムスタンプ"=w571, "Value"=w569) -> (".NET refnum出力"=w565:refnum<k24>)  [unwired: 5 in, 1 out]
                    n324 = call "LC-MISDK_UserCalibration_MakeListData_XYZ.vi"("Before_2"=w575, "Before_3"=w570, "before_1"=w576, "タイムスタンプ"=w571, "Value"=w569) -> (".NET refnum出力"=w564:refnum<k24>)  [unwired: 5 in, 1 out]
                  }
                }
                n325 = invoke on="インボークノード" class="List`1[[Konicaminolta.XYZ, LC-M" method="Add"(reference=w558, "item"=w562) -> (reference out=w556:refnum<k24>)  [unwired: 2 in, 3 out]
                n326 = invoke on="インボークノード" class="List`1[[Konicaminolta.XYZ, LC-M" method="Add"(reference=w556, "item"=w557) -> (reference out=w554:refnum<k24>)  [unwired: 2 in, 3 out]
                n327 = invoke on="インボークノード" class="List`1[[Konicaminolta.XYZ, LC-M" method="Add"(reference=w554, "item"=w555) -> (reference out=w549:refnum<k24>)  [unwired: 2 in, 3 out]
                n328 = invoke on="インボークノード" class="List`1[[Konicaminolta.XYZ, LC-M" method="Add"(reference=w559, "item"=w560) -> (reference out=w553:refnum<k24>)  [unwired: 2 in, 3 out]
                n329 = invoke on="インボークノード" class="List`1[[Konicaminolta.XYZ, LC-M" method="Add"(reference=w553, "item"=w552) -> (reference out=w551:refnum<k24>)  [unwired: 2 in, 3 out]
                n330 = invoke on="インボークノード" class="List`1[[Konicaminolta.XYZ, LC-M" method="Add"(reference=w551, "item"=w550) -> (reference out=w548:refnum<k24>)  [unwired: 2 in, 3 out]
              }
              frame "WRGB" {
                n331 = flat-sequence {
                  tunnel: w617 -> [w620]
                  tunnel: [w655] -> w616
                  tunnel: w615 -> [w623]
                  tunnel: [w636] -> w614
                  tunnel: [w635] -> w612
                  tunnel: [w629] -> w607
                  tunnel: [w628] -> w606
                  tunnel: [w627] -> w604
                  tunnel: [w626] -> w603
                  tunnel: [w625] -> w602
                  tunnel: [w619] -> w601
                  tunnel: [w618] -> w600
                  frame #0 {
                    n332 = property on="After_R" class="Clust （指定）"() -> ("Value"=w653:T3)  [unwired: 2 in, 2 out]
                    n333 = property on="After_B" class="Clust （指定）"() -> ("Value"=w639:T1)  [unwired: 2 in, 2 out]
                    n334 = property on="After_G" class="Clust （指定）"() -> ("Value"=w637:T2)  [unwired: 2 in, 2 out]
                    n335 = property on="Before_W" class="Clust （指定）"() -> ("Value"=w634:T8)  [unwired: 2 in, 2 out]
                    n336 = property on="Before_R" class="Clust （指定）"() -> ("Value"=w654:T7)  [unwired: 2 in, 2 out]
                    n337 = property on="Before_G" class="Clust （指定）"() -> ("Value"=w649:T6)  [unwired: 2 in, 2 out]
                    n338 = property on="Before_B" class="Clust （指定）"() -> ("Value"=w645:T5)  [unwired: 2 in, 2 out]
                    n339 = property on="After_W" class="Clust （指定）"() -> ("Value"=w630:T4)  [unwired: 2 in, 2 out]
                    n340 = Unbundle(w653) -> ("After_R1"=w658:dbl, "After_R2"=w657:dbl, "After_R3"=w656:dbl)
                    n341 = Unbundle(w637) -> ("After_G1"=w644:dbl, "After_G2"=w643:dbl, "After_G3"=w642:dbl)
                    n342 = Unbundle(w639) -> ("After_B1"=w641:dbl, "After_B2"=w640:dbl, "After_B3"=w638:dbl)
                    n343 = Unbundle(w634) -> ("before_W1"=w622:dbl, "Before_W2"=w624:dbl, "Before_W3"=w621:dbl)
                    n344 = Unbundle(w654) -> ("before_R1"=w661:dbl, "Before_R2"=w660:dbl, "Before_R3"=w659:dbl)
                    n345 = Unbundle(w649) -> ("before_G1"=w652:dbl, "Before_G2"=w651:dbl, "Before_G3"=w650:dbl)
                    n346 = Unbundle(w630) -> ("After_W1"=w631:dbl, "After_W2"=w632:dbl, "After_W3"=w633:dbl)
                    n347 = Unbundle(w645) -> ("before_B1"=w648:dbl, "Before_B2"=w647:dbl, "Before_B3"=w646:dbl)
                    n348 = call "LC-MISDK_UserCalibration_MakeListData_XYZ.vi"("Before_2"=w660, "Before_3"=w659, "before_1"=w661, "タイムスタンプ"=w623, "Value"=w620) -> (".NET refnum出力"=w655:refnum<k24>)  [unwired: 5 in, 1 out]
                    n349 = call "LC-MISDK_UserCalibration_MakeListData_XYZ.vi"("Before_2"=w624, "Before_3"=w621, "before_1"=w622, "タイムスタンプ"=w623, "Value"=w620) -> ("リファレンス出力"=w618:refnum<k24>, ".NET refnum出力"=w619:refnum<k24>)  [unwired: 5 in]
                    n350 = call "LC-MISDK_UserCalibration_MakeListData_XYZ.vi"("Before_2"=w651, "Before_3"=w650, "before_1"=w652, "タイムスタンプ"=w623, "Value"=w620) -> (".NET refnum出力"=w636:refnum<k24>)  [unwired: 5 in, 1 out]
                    n351 = call "LC-MISDK_UserCalibration_MakeListData_XYZ.vi"("Before_2"=w657, "Before_3"=w656, "before_1"=w658, "タイムスタンプ"=w623, "Value"=w620) -> (".NET refnum出力"=w627:refnum<k24>)  [unwired: 5 in, 1 out]
                    n352 = call "LC-MISDK_UserCalibration_MakeListData_XYZ.vi"("Before_2"=w632, "Before_3"=w633, "before_1"=w631, "タイムスタンプ"=w623, "Value"=w620) -> ("リファレンス出力"=w628:refnum<k24>, ".NET refnum出力"=w629:refnum<k24>)  [unwired: 5 in]
                    n353 = call "LC-MISDK_UserCalibration_MakeListData_XYZ.vi"("Before_2"=w647, "Before_3"=w646, "before_1"=w648, "タイムスタンプ"=w623, "Value"=w620) -> (".NET refnum出力"=w635:refnum<k24>)  [unwired: 5 in, 1 out]
                    n354 = call "LC-MISDK_UserCalibration_MakeListData_XYZ.vi"("Before_2"=w643, "Before_3"=w642, "before_1"=w644, "タイムスタンプ"=w623, "Value"=w620) -> (".NET refnum出力"=w626:refnum<k24>)  [unwired: 5 in, 1 out]
                    n355 = call "LC-MISDK_UserCalibration_MakeListData_XYZ.vi"("Before_2"=w640, "Before_3"=w638, "before_1"=w641, "タイムスタンプ"=w623, "Value"=w620) -> (".NET refnum出力"=w625:refnum<k24>)  [unwired: 5 in, 1 out]
                  }
                }
                n356 = invoke on="インボークノード" class="List`1[[Konicaminolta.XYZ, LC-M" method="Add"(reference=w606, "item"=w607) -> (reference out=w605:refnum<k24>)  [unwired: 2 in, 3 out]
                n357 = invoke on="インボークノード" class="List`1[[Konicaminolta.XYZ, LC-M" method="Add"(reference=w600, "item"=w601) -> (reference out=w608:refnum<k24>)  [unwired: 2 in, 3 out]
                n358 = invoke on="インボークノード" class="List`1[[Konicaminolta.XYZ, LC-M" method="Add"(reference=w608, "item"=w616) -> (reference out=w613:refnum<k24>)  [unwired: 2 in, 3 out]
                n359 = invoke on="インボークノード" class="List`1[[Konicaminolta.XYZ, LC-M" method="Add"(reference=w613, "item"=w614) -> (reference out=w611:refnum<k24>)  [unwired: 2 in, 3 out]
                n360 = invoke on="インボークノード" class="List`1[[Konicaminolta.XYZ, LC-M" method="Add"(reference=w611, "item"=w612) -> (reference out=w599:refnum<k24>)  [unwired: 2 in, 3 out]
                n361 = invoke on="インボークノード" class="List`1[[Konicaminolta.XYZ, LC-M" method="Add"(reference=w605, "item"=w604) -> (reference out=w610:refnum<k24>)  [unwired: 2 in, 3 out]
                n362 = invoke on="インボークノード" class="List`1[[Konicaminolta.XYZ, LC-M" method="Add"(reference=w610, "item"=w603) -> (reference out=w609:refnum<k24>)  [unwired: 2 in, 3 out]
                n363 = invoke on="インボークノード" class="List`1[[Konicaminolta.XYZ, LC-M" method="Add"(reference=w609, "item"=w602) -> (reference out=w598:refnum<k24>)  [unwired: 2 in, 3 out]
              }
            }
            n364 = invoke on="インボークノード" class="LightColorMISDK" method="SetMatrixCalib"(reference=w525, "calibrationCh"=w524, "measurementDataList"=w515, "correctDataList"=w514, "type"=w516, "id"=w523, "comPort"=0) -> (error out=w521:errorcluster, "SetMatrixCalib"=w522:refnum<k24>)  [unwired: 2 in, 7 out]
            n365 = property on="プロパティノード" class="ReturnMessage"(reference=w522, error in=w521) -> (error out=w520:errorcluster, "errorCode"=w513:i32)  [unwired: 1 out]
            n366 = property on="error out" class="Clust （指定）"("Value"=w520) -> ()  [unwired: 2 in, 2 out]
            n367 = property on="CalError" class="DigNum （指定）"("Value"=w513) -> ()  [unwired: 2 in, 2 out]
          }
          frame "Lv,λd,Pe" {
            n368 = case shown="\"Single-Point\", デフォルト" w665 {
              tunnel: w667 -> [w682 w712 w766]
              tunnel: [w681 w698 w748] -> w664
              tunnel: [w679 w697 w747] -> w663
              tunnel: w666 -> [w675 w710 w764]
              frame "Single-Point", Default {
                n369 = flat-sequence {
                  tunnel: w682 -> [w691]
                  tunnel: [w687] -> w680
                  tunnel: [w686] -> w678
                  tunnel: [w685] -> w677
                  tunnel: [w684] -> w676
                  tunnel: w675 -> [w683]
                  frame #0 {
                    n370 = property on="After_W" class="Clust （指定）"() -> ("Value"=w695:T4)  [unwired: 2 in, 2 out]
                    n371 = Unbundle(w695) -> ("After_W1"=w690:dbl, "After_W2"=w689:dbl, "After_W3"=w688:dbl)
                    n372 = property on="Before_W" class="Clust （指定）"() -> ("Value"=w696:T8)  [unwired: 2 in, 2 out]
                    n373 = Unbundle(w696) -> ("before_W1"=w694:dbl, "Before_W2"=w693:dbl, "Before_W3"=w692:dbl)
                    n374 = call "LC-MISDK_UserCalibration_MakeListData_LvλdPe.vi"("Before_2"=w689, "Before_3"=w688, "before_1"=w690, "タイムスタンプ"=w683, "Value"=w691) -> ("リファレンス出力"=w686:refnum<k24>, ".NET refnum出力"=w687:refnum<k24>)  [unwired: 5 in]
                    n375 = call "LC-MISDK_UserCalibration_MakeListData_LvλdPe.vi"("Before_2"=w693, "Before_3"=w692, "before_1"=w694, "タイムスタンプ"=w683, "Value"=w691) -> ("リファレンス出力"=w684:refnum<k24>, ".NET refnum出力"=w685:refnum<k24>)  [unwired: 5 in]
                  }
                }
                n376 = invoke on="インボークノード" class="List`1[[Konicaminolta.LvDwPe, L" method="Add"(reference=w676, "item"=w677) -> (reference out=w681:refnum<k24>)  [unwired: 2 in, 3 out]
                n377 = invoke on="インボークノード" class="List`1[[Konicaminolta.LvDwPe, L" method="Add"(reference=w678, "item"=w680) -> (reference out=w679:refnum<k24>)  [unwired: 2 in, 3 out]
              }
              frame "RGB" {
                n378 = flat-sequence {
                  tunnel: w712 -> [w718]
                  tunnel: [w740] -> w711
                  tunnel: [w739] -> w707
                  tunnel: w710 -> [w720]
                  tunnel: [w723] -> w709
                  tunnel: [w722] -> w708
                  tunnel: [w716] -> w706
                  tunnel: [w715] -> w704
                  tunnel: [w714] -> w701
                  tunnel: [w713] -> w699
                  frame #0 {
                    n379 = property on="After_R" class="Clust （指定）"() -> ("Value"=w737:T3)  [unwired: 2 in, 2 out]
                    n380 = property on="After_B" class="Clust （指定）"() -> ("Value"=w721:T1)  [unwired: 2 in, 2 out]
                    n381 = property on="After_G" class="Clust （指定）"() -> ("Value"=w717:T2)  [unwired: 2 in, 2 out]
                    n382 = property on="Before_R" class="Clust （指定）"() -> ("Value"=w738:T7)  [unwired: 2 in, 2 out]
                    n383 = property on="Before_G" class="Clust （指定）"() -> ("Value"=w733:T6)  [unwired: 2 in, 2 out]
                    n384 = property on="Before_B" class="Clust （指定）"() -> ("Value"=w729:T5)  [unwired: 2 in, 2 out]
                    n385 = Unbundle(w737) -> ("After_R1"=w743:dbl, "After_R2"=w742:dbl, "After_R3"=w741:dbl)
                    n386 = Unbundle(w717) -> ("After_G1"=w728:dbl, "After_G2"=w727:dbl, "After_G3"=w726:dbl)
                    n387 = Unbundle(w721) -> ("After_B1"=w725:dbl, "After_B2"=w724:dbl, "After_B3"=w719:dbl)
                    n388 = Unbundle(w738) -> ("before_R1"=w746:dbl, "Before_R2"=w745:dbl, "Before_R3"=w744:dbl)
                    n389 = Unbundle(w733) -> ("before_G1"=w736:dbl, "Before_G2"=w735:dbl, "Before_G3"=w734:dbl)
                    n390 = Unbundle(w729) -> ("before_B1"=w732:dbl, "Before_B2"=w731:dbl, "Before_B3"=w730:dbl)
                    n391 = call "LC-MISDK_UserCalibration_MakeListData_LvλdPe.vi"("Before_2"=w745, "Before_3"=w744, "before_1"=w746, "タイムスタンプ"=w720, "Value"=w718) -> ("リファレンス出力"=w739:refnum<k24>, ".NET refnum出力"=w740:refnum<k24>)  [unwired: 5 in]
                    n392 = call "LC-MISDK_UserCalibration_MakeListData_LvλdPe.vi"("Before_2"=w735, "Before_3"=w734, "before_1"=w736, "タイムスタンプ"=w720, "Value"=w718) -> (".NET refnum出力"=w716:refnum<k24>)  [unwired: 5 in, 1 out]
                    n393 = call "LC-MISDK_UserCalibration_MakeListData_LvλdPe.vi"("Before_2"=w742, "Before_3"=w741, "before_1"=w743, "タイムスタンプ"=w720, "Value"=w718) -> ("リファレンス出力"=w722:refnum<k24>, ".NET refnum出力"=w723:refnum<k24>)  [unwired: 5 in]
                    n394 = call "LC-MISDK_UserCalibration_MakeListData_LvλdPe.vi"("Before_2"=w731, "Before_3"=w730, "before_1"=w732, "タイムスタンプ"=w720, "Value"=w718) -> (".NET refnum出力"=w715:refnum<k24>)  [unwired: 5 in, 1 out]
                    n395 = call "LC-MISDK_UserCalibration_MakeListData_LvλdPe.vi"("Before_2"=w727, "Before_3"=w726, "before_1"=w728, "タイムスタンプ"=w720, "Value"=w718) -> (".NET refnum出力"=w714:refnum<k24>)  [unwired: 5 in, 1 out]
                    n396 = call "LC-MISDK_UserCalibration_MakeListData_LvλdPe.vi"("Before_2"=w724, "Before_3"=w719, "before_1"=w725, "タイムスタンプ"=w720, "Value"=w718) -> (".NET refnum出力"=w713:refnum<k24>)  [unwired: 5 in, 1 out]
                  }
                }
                n397 = invoke on="インボークノード" class="List`1[[Konicaminolta.LvDwPe, L" method="Add"(reference=w707, "item"=w711) -> (reference out=w705:refnum<k24>)  [unwired: 2 in, 3 out]
                n398 = invoke on="インボークノード" class="List`1[[Konicaminolta.LvDwPe, L" method="Add"(reference=w705, "item"=w706) -> (reference out=w703:refnum<k24>)  [unwired: 2 in, 3 out]
                n399 = invoke on="インボークノード" class="List`1[[Konicaminolta.LvDwPe, L" method="Add"(reference=w703, "item"=w704) -> (reference out=w698:refnum<k24>)  [unwired: 2 in, 3 out]
                n400 = invoke on="インボークノード" class="List`1[[Konicaminolta.LvDwPe, L" method="Add"(reference=w708, "item"=w709) -> (reference out=w702:refnum<k24>)  [unwired: 2 in, 3 out]
                n401 = invoke on="インボークノード" class="List`1[[Konicaminolta.LvDwPe, L" method="Add"(reference=w702, "item"=w701) -> (reference out=w700:refnum<k24>)  [unwired: 2 in, 3 out]
                n402 = invoke on="インボークノード" class="List`1[[Konicaminolta.LvDwPe, L" method="Add"(reference=w700, "item"=w699) -> (reference out=w697:refnum<k24>)  [unwired: 2 in, 3 out]
              }
              frame "WRGB" {
                n403 = flat-sequence {
                  tunnel: w766 -> [w769]
                  tunnel: [w804] -> w765
                  tunnel: w764 -> [w772]
                  tunnel: [w785] -> w763
                  tunnel: [w784] -> w761
                  tunnel: [w778] -> w756
                  tunnel: [w777] -> w755
                  tunnel: [w776] -> w753
                  tunnel: [w775] -> w752
                  tunnel: [w774] -> w751
                  tunnel: [w768] -> w750
                  tunnel: [w767] -> w749
                  frame #0 {
                    n404 = property on="After_R" class="Clust （指定）"() -> ("Value"=w802:T3)  [unwired: 2 in, 2 out]
                    n405 = property on="After_B" class="Clust （指定）"() -> ("Value"=w788:T1)  [unwired: 2 in, 2 out]
                    n406 = property on="After_G" class="Clust （指定）"() -> ("Value"=w786:T2)  [unwired: 2 in, 2 out]
                    n407 = property on="Before_W" class="Clust （指定）"() -> ("Value"=w783:T8)  [unwired: 2 in, 2 out]
                    n408 = property on="Before_R" class="Clust （指定）"() -> ("Value"=w803:T7)  [unwired: 2 in, 2 out]
                    n409 = property on="Before_G" class="Clust （指定）"() -> ("Value"=w798:T6)  [unwired: 2 in, 2 out]
                    n410 = property on="Before_B" class="Clust （指定）"() -> ("Value"=w794:T5)  [unwired: 2 in, 2 out]
                    n411 = property on="After_W" class="Clust （指定）"() -> ("Value"=w779:T4)  [unwired: 2 in, 2 out]
                    n412 = Unbundle(w802) -> ("After_R1"=w807:dbl, "After_R2"=w806:dbl, "After_R3"=w805:dbl)
                    n413 = Unbundle(w786) -> ("After_G1"=w793:dbl, "After_G2"=w792:dbl, "After_G3"=w791:dbl)
                    n414 = Unbundle(w788) -> ("After_B1"=w790:dbl, "After_B2"=w789:dbl, "After_B3"=w787:dbl)
                    n415 = Unbundle(w783) -> ("before_W1"=w771:dbl, "Before_W2"=w773:dbl, "Before_W3"=w770:dbl)
                    n416 = Unbundle(w803) -> ("before_R1"=w810:dbl, "Before_R2"=w809:dbl, "Before_R3"=w808:dbl)
                    n417 = Unbundle(w798) -> ("before_G1"=w801:dbl, "Before_G2"=w800:dbl, "Before_G3"=w799:dbl)
                    n418 = Unbundle(w779) -> ("After_W1"=w780:dbl, "After_W2"=w781:dbl, "After_W3"=w782:dbl)
                    n419 = Unbundle(w794) -> ("before_B1"=w797:dbl, "Before_B2"=w796:dbl, "Before_B3"=w795:dbl)
                    n420 = call "LC-MISDK_UserCalibration_MakeListData_LvλdPe.vi"("Before_2"=w809, "Before_3"=w808, "before_1"=w810, "タイムスタンプ"=w772, "Value"=w769) -> (".NET refnum出力"=w804:refnum<k24>)  [unwired: 5 in, 1 out]
                    n421 = call "LC-MISDK_UserCalibration_MakeListData_LvλdPe.vi"("Before_2"=w773, "Before_3"=w770, "before_1"=w771, "タイムスタンプ"=w772, "Value"=w769) -> ("リファレンス出力"=w767:refnum<k24>, ".NET refnum出力"=w768:refnum<k24>)  [unwired: 5 in]
                    n422 = call "LC-MISDK_UserCalibration_MakeListData_LvλdPe.vi"("Before_2"=w800, "Before_3"=w799, "before_1"=w801, "タイムスタンプ"=w772, "Value"=w769) -> (".NET refnum出力"=w785:refnum<k24>)  [unwired: 5 in, 1 out]
                    n423 = call "LC-MISDK_UserCalibration_MakeListData_LvλdPe.vi"("Before_2"=w806, "Before_3"=w805, "before_1"=w807, "タイムスタンプ"=w772, "Value"=w769) -> (".NET refnum出力"=w776:refnum<k24>)  [unwired: 5 in, 1 out]
                    n424 = call "LC-MISDK_UserCalibration_MakeListData_LvλdPe.vi"("Before_2"=w781, "Before_3"=w782, "before_1"=w780, "タイムスタンプ"=w772, "Value"=w769) -> ("リファレンス出力"=w777:refnum<k24>, ".NET refnum出力"=w778:refnum<k24>)  [unwired: 5 in]
                    n425 = call "LC-MISDK_UserCalibration_MakeListData_LvλdPe.vi"("Before_2"=w796, "Before_3"=w795, "before_1"=w797, "タイムスタンプ"=w772, "Value"=w769) -> (".NET refnum出力"=w784:refnum<k24>)  [unwired: 5 in, 1 out]
                    n426 = call "LC-MISDK_UserCalibration_MakeListData_LvλdPe.vi"("Before_2"=w792, "Before_3"=w791, "before_1"=w793, "タイムスタンプ"=w772, "Value"=w769) -> (".NET refnum出力"=w775:refnum<k24>)  [unwired: 5 in, 1 out]
                    n427 = call "LC-MISDK_UserCalibration_MakeListData_LvλdPe.vi"("Before_2"=w789, "Before_3"=w787, "before_1"=w790, "タイムスタンプ"=w772, "Value"=w769) -> (".NET refnum出力"=w774:refnum<k24>)  [unwired: 5 in, 1 out]
                  }
                }
                n428 = invoke on="インボークノード" class="List`1[[Konicaminolta.LvDwPe, L" method="Add"(reference=w755, "item"=w756) -> (reference out=w754:refnum<k24>)  [unwired: 2 in, 3 out]
                n429 = invoke on="インボークノード" class="List`1[[Konicaminolta.LvDwPe, L" method="Add"(reference=w749, "item"=w750) -> (reference out=w757:refnum<k24>)  [unwired: 2 in, 3 out]
                n430 = invoke on="インボークノード" class="List`1[[Konicaminolta.LvDwPe, L" method="Add"(reference=w757, "item"=w765) -> (reference out=w762:refnum<k24>)  [unwired: 2 in, 3 out]
                n431 = invoke on="インボークノード" class="List`1[[Konicaminolta.LvDwPe, L" method="Add"(reference=w762, "item"=w763) -> (reference out=w760:refnum<k24>)  [unwired: 2 in, 3 out]
                n432 = invoke on="インボークノード" class="List`1[[Konicaminolta.LvDwPe, L" method="Add"(reference=w760, "item"=w761) -> (reference out=w748:refnum<k24>)  [unwired: 2 in, 3 out]
                n433 = invoke on="インボークノード" class="List`1[[Konicaminolta.LvDwPe, L" method="Add"(reference=w754, "item"=w753) -> (reference out=w759:refnum<k24>)  [unwired: 2 in, 3 out]
                n434 = invoke on="インボークノード" class="List`1[[Konicaminolta.LvDwPe, L" method="Add"(reference=w759, "item"=w752) -> (reference out=w758:refnum<k24>)  [unwired: 2 in, 3 out]
                n435 = invoke on="インボークノード" class="List`1[[Konicaminolta.LvDwPe, L" method="Add"(reference=w758, "item"=w751) -> (reference out=w747:refnum<k24>)  [unwired: 2 in, 3 out]
              }
            }
            n436 = invoke on="インボークノード" class="LightColorMISDK" method="SetMatrixCalib"(reference=w674, "calibrationCh"=w673, "measurementDataList"=w664, "correctDataList"=w663, "type"=w665, "id"=w672, "comPort"=0) -> (error out=w670:errorcluster, "SetMatrixCalib"=w671:refnum<k24>)  [unwired: 2 in, 7 out]
            n437 = property on="プロパティノード" class="ReturnMessage"(reference=w671, error in=w670) -> (error out=w669:errorcluster, "errorCode"=w662:i32)  [unwired: 1 out]
            n438 = property on="error out" class="Clust （指定）"("Value"=w669) -> ()  [unwired: 2 in, 2 out]
            n439 = property on="CalError" class="DigNum （指定）"("Value"=w662) -> ()  [unwired: 2 in, 2 out]
          }
          frame "Lv,x,y", Default {
            (unwired) refnum<k24> refnum ("リファレンス出力")
            n440 = case shown="\"Single-Point\", デフォルト" w814 {
              tunnel: w816 -> [w831 w861 w915]
              tunnel: [w830 w847 w897] -> w813
              tunnel: [w828 w846 w896] -> w812
              tunnel: w815 -> [w824 w859 w913]
              frame "Single-Point", Default {
                n441 = flat-sequence {
                  tunnel: w831 -> [w840]
                  tunnel: [w836] -> w829
                  tunnel: [w835] -> w827
                  tunnel: [w834] -> w826
                  tunnel: [w833] -> w825
                  tunnel: w824 -> [w832]
                  frame #0 {
                    n442 = property on="After_W" class="Clust （指定）"() -> ("Value"=w844:T4)  [unwired: 2 in, 2 out]
                    n443 = Unbundle(w844) -> ("After_W1"=w839:dbl, "After_W2"=w838:dbl, "After_W3"=w837:dbl)
                    n444 = property on="Before_W" class="Clust （指定）"() -> ("Value"=w845:T8)  [unwired: 2 in, 2 out]
                    n445 = Unbundle(w845) -> ("before_W1"=w843:dbl, "Before_W2"=w842:dbl, "Before_W3"=w841:dbl)
                    n446 = call "LC-MISDK_UserCalibration_MakeListData_Lvx.vi"("Before_2"=w838, "Before_3"=w837, "before_1"=w839, "タイムスタンプ"=w832, "Value"=w840) -> ("リファレンス出力"=w835:refnum<k24>, ".NET refnum出力"=w836:refnum<k24>)  [unwired: 5 in]
                    n447 = call "LC-MISDK_UserCalibration_MakeListData_Lvx.vi"("Before_2"=w842, "Before_3"=w841, "before_1"=w843, "タイムスタンプ"=w832, "Value"=w840) -> ("リファレンス出力"=w833:refnum<k24>, ".NET refnum出力"=w834:refnum<k24>)  [unwired: 5 in]
                  }
                }
                n448 = invoke on="インボークノード" class="List`1[[Konicaminolta.Lvxy, LC-" method="Add"(reference=w825, "item"=w826) -> (reference out=w830:refnum<k24>)  [unwired: 2 in, 3 out]
                n449 = invoke on="インボークノード" class="List`1[[Konicaminolta.Lvxy, LC-" method="Add"(reference=w827, "item"=w829) -> (reference out=w828:refnum<k24>)  [unwired: 2 in, 3 out]
              }
              frame "RGB" {
                n450 = flat-sequence {
                  tunnel: w861 -> [w867]
                  tunnel: [w889] -> w860
                  tunnel: [w888] -> w856
                  tunnel: w859 -> [w869]
                  tunnel: [w872] -> w858
                  tunnel: [w871] -> w857
                  tunnel: [w865] -> w855
                  tunnel: [w864] -> w853
                  tunnel: [w863] -> w850
                  tunnel: [w862] -> w848
                  frame #0 {
                    n451 = property on="After_R" class="Clust （指定）"() -> ("Value"=w886:T3)  [unwired: 2 in, 2 out]
                    n452 = property on="After_B" class="Clust （指定）"() -> ("Value"=w870:T1)  [unwired: 2 in, 2 out]
                    n453 = property on="After_G" class="Clust （指定）"() -> ("Value"=w866:T2)  [unwired: 2 in, 2 out]
                    n454 = property on="Before_R" class="Clust （指定）"() -> ("Value"=w887:T7)  [unwired: 2 in, 2 out]
                    n455 = property on="Before_G" class="Clust （指定）"() -> ("Value"=w882:T6)  [unwired: 2 in, 2 out]
                    n456 = property on="Before_B" class="Clust （指定）"() -> ("Value"=w878:T5)  [unwired: 2 in, 2 out]
                    n457 = Unbundle(w886) -> ("After_R1"=w892:dbl, "After_R2"=w891:dbl, "After_R3"=w890:dbl)
                    n458 = Unbundle(w866) -> ("After_G1"=w877:dbl, "After_G2"=w876:dbl, "After_G3"=w875:dbl)
                    n459 = Unbundle(w870) -> ("After_B1"=w874:dbl, "After_B2"=w873:dbl, "After_B3"=w868:dbl)
                    n460 = Unbundle(w887) -> ("before_R1"=w895:dbl, "Before_R2"=w894:dbl, "Before_R3"=w893:dbl)
                    n461 = Unbundle(w882) -> ("before_G1"=w885:dbl, "Before_G2"=w884:dbl, "Before_G3"=w883:dbl)
                    n462 = Unbundle(w878) -> ("before_B1"=w881:dbl, "Before_B2"=w880:dbl, "Before_B3"=w879:dbl)
                    n463 = call "LC-MISDK_UserCalibration_MakeListData_Lvx.vi"("Before_2"=w894, "Before_3"=w893, "before_1"=w895, "タイムスタンプ"=w869, "Value"=w867) -> ("リファレンス出力"=w888:refnum<k24>, ".NET refnum出力"=w889:refnum<k24>)  [unwired: 5 in]
                    n464 = call "LC-MISDK_UserCalibration_MakeListData_Lvx.vi"("Before_2"=w884, "Before_3"=w883, "before_1"=w885, "タイムスタンプ"=w869, "Value"=w867) -> (".NET refnum出力"=w865:refnum<k24>)  [unwired: 5 in, 1 out]
                    n465 = call "LC-MISDK_UserCalibration_MakeListData_Lvx.vi"("Before_2"=w891, "Before_3"=w890, "before_1"=w892, "タイムスタンプ"=w869, "Value"=w867) -> ("リファレンス出力"=w871:refnum<k24>, ".NET refnum出力"=w872:refnum<k24>)  [unwired: 5 in]
                    n466 = call "LC-MISDK_UserCalibration_MakeListData_Lvx.vi"("Before_2"=w880, "Before_3"=w879, "before_1"=w881, "タイムスタンプ"=w869, "Value"=w867) -> (".NET refnum出力"=w864:refnum<k24>)  [unwired: 5 in, 1 out]
                    n467 = call "LC-MISDK_UserCalibration_MakeListData_Lvx.vi"("Before_2"=w876, "Before_3"=w875, "before_1"=w877, "タイムスタンプ"=w869, "Value"=w867) -> (".NET refnum出力"=w863:refnum<k24>)  [unwired: 5 in, 1 out]
                    n468 = call "LC-MISDK_UserCalibration_MakeListData_Lvx.vi"("Before_2"=w873, "Before_3"=w868, "before_1"=w874, "タイムスタンプ"=w869, "Value"=w867) -> (".NET refnum出力"=w862:refnum<k24>)  [unwired: 5 in, 1 out]
                  }
                }
                n469 = invoke on="インボークノード" class="List`1[[Konicaminolta.Lvxy, LC-" method="Add"(reference=w856, "item"=w860) -> (reference out=w854:refnum<k24>)  [unwired: 2 in, 3 out]
                n470 = invoke on="インボークノード" class="List`1[[Konicaminolta.Lvxy, LC-" method="Add"(reference=w854, "item"=w855) -> (reference out=w852:refnum<k24>)  [unwired: 2 in, 3 out]
                n471 = invoke on="インボークノード" class="List`1[[Konicaminolta.Lvxy, LC-" method="Add"(reference=w852, "item"=w853) -> (reference out=w847:refnum<k24>)  [unwired: 2 in, 3 out]
                n472 = invoke on="インボークノード" class="List`1[[Konicaminolta.Lvxy, LC-" method="Add"(reference=w857, "item"=w858) -> (reference out=w851:refnum<k24>)  [unwired: 2 in, 3 out]
                n473 = invoke on="インボークノード" class="List`1[[Konicaminolta.Lvxy, LC-" method="Add"(reference=w851, "item"=w850) -> (reference out=w849:refnum<k24>)  [unwired: 2 in, 3 out]
                n474 = invoke on="インボークノード" class="List`1[[Konicaminolta.Lvxy, LC-" method="Add"(reference=w849, "item"=w848) -> (reference out=w846:refnum<k24>)  [unwired: 2 in, 3 out]
              }
              frame "WRGB" {
                n475 = flat-sequence {
                  tunnel: w915 -> [w918]
                  tunnel: [w953] -> w914
                  tunnel: w913 -> [w921]
                  tunnel: [w934] -> w912
                  tunnel: [w933] -> w910
                  tunnel: [w927] -> w905
                  tunnel: [w926] -> w904
                  tunnel: [w925] -> w902
                  tunnel: [w924] -> w901
                  tunnel: [w923] -> w900
                  tunnel: [w917] -> w899
                  tunnel: [w916] -> w898
                  frame #0 {
                    n476 = property on="After_R" class="Clust （指定）"() -> ("Value"=w951:T3)  [unwired: 2 in, 2 out]
                    n477 = property on="After_B" class="Clust （指定）"() -> ("Value"=w937:T1)  [unwired: 2 in, 2 out]
                    n478 = property on="After_G" class="Clust （指定）"() -> ("Value"=w935:T2)  [unwired: 2 in, 2 out]
                    n479 = property on="Before_W" class="Clust （指定）"() -> ("Value"=w932:T8)  [unwired: 2 in, 2 out]
                    n480 = property on="Before_R" class="Clust （指定）"() -> ("Value"=w952:T7)  [unwired: 2 in, 2 out]
                    n481 = property on="Before_G" class="Clust （指定）"() -> ("Value"=w947:T6)  [unwired: 2 in, 2 out]
                    n482 = property on="Before_B" class="Clust （指定）"() -> ("Value"=w943:T5)  [unwired: 2 in, 2 out]
                    n483 = property on="After_W" class="Clust （指定）"() -> ("Value"=w928:T4)  [unwired: 2 in, 2 out]
                    n484 = Unbundle(w951) -> ("After_R1"=w956:dbl, "After_R2"=w955:dbl, "After_R3"=w954:dbl)
                    n485 = Unbundle(w935) -> ("After_G1"=w942:dbl, "After_G2"=w941:dbl, "After_G3"=w940:dbl)
                    n486 = Unbundle(w937) -> ("After_B1"=w939:dbl, "After_B2"=w938:dbl, "After_B3"=w936:dbl)
                    n487 = Unbundle(w932) -> ("before_W1"=w920:dbl, "Before_W2"=w922:dbl, "Before_W3"=w919:dbl)
                    n488 = Unbundle(w952) -> ("before_R1"=w959:dbl, "Before_R2"=w958:dbl, "Before_R3"=w957:dbl)
                    n489 = Unbundle(w947) -> ("before_G1"=w950:dbl, "Before_G2"=w949:dbl, "Before_G3"=w948:dbl)
                    n490 = Unbundle(w928) -> ("After_W1"=w929:dbl, "After_W2"=w930:dbl, "After_W3"=w931:dbl)
                    n491 = Unbundle(w943) -> ("before_B1"=w946:dbl, "Before_B2"=w945:dbl, "Before_B3"=w944:dbl)
                    n492 = call "LC-MISDK_UserCalibration_MakeListData_Lvx.vi"("Before_2"=w958, "Before_3"=w957, "before_1"=w959, "タイムスタンプ"=w921, "Value"=w918) -> (".NET refnum出力"=w953:refnum<k24>)  [unwired: 5 in, 1 out]
                    n493 = call "LC-MISDK_UserCalibration_MakeListData_Lvx.vi"("Before_2"=w922, "Before_3"=w919, "before_1"=w920, "タイムスタンプ"=w921, "Value"=w918) -> ("リファレンス出力"=w916:refnum<k24>, ".NET refnum出力"=w917:refnum<k24>)  [unwired: 5 in]
                    n494 = call "LC-MISDK_UserCalibration_MakeListData_Lvx.vi"("Before_2"=w949, "Before_3"=w948, "before_1"=w950, "タイムスタンプ"=w921, "Value"=w918) -> (".NET refnum出力"=w934:refnum<k24>)  [unwired: 5 in, 1 out]
                    n495 = call "LC-MISDK_UserCalibration_MakeListData_Lvx.vi"("Before_2"=w955, "Before_3"=w954, "before_1"=w956, "タイムスタンプ"=w921, "Value"=w918) -> (".NET refnum出力"=w925:refnum<k24>)  [unwired: 5 in, 1 out]
                    n496 = call "LC-MISDK_UserCalibration_MakeListData_Lvx.vi"("Before_2"=w930, "Before_3"=w931, "before_1"=w929, "タイムスタンプ"=w921, "Value"=w918) -> ("リファレンス出力"=w926:refnum<k24>, ".NET refnum出力"=w927:refnum<k24>)  [unwired: 5 in]
                    n497 = call "LC-MISDK_UserCalibration_MakeListData_Lvx.vi"("Before_2"=w945, "Before_3"=w944, "before_1"=w946, "タイムスタンプ"=w921, "Value"=w918) -> (".NET refnum出力"=w933:refnum<k24>)  [unwired: 5 in, 1 out]
                    n498 = call "LC-MISDK_UserCalibration_MakeListData_Lvx.vi"("Before_2"=w941, "Before_3"=w940, "before_1"=w942, "タイムスタンプ"=w921, "Value"=w918) -> (".NET refnum出力"=w924:refnum<k24>)  [unwired: 5 in, 1 out]
                    n499 = call "LC-MISDK_UserCalibration_MakeListData_Lvx.vi"("Before_2"=w938, "Before_3"=w936, "before_1"=w939, "タイムスタンプ"=w921, "Value"=w918) -> (".NET refnum出力"=w923:refnum<k24>)  [unwired: 5 in, 1 out]
                  }
                }
                n500 = invoke on="インボークノード" class="List`1[[Konicaminolta.Lvxy, LC-" method="Add"(reference=w904, "item"=w905) -> (reference out=w903:refnum<k24>)  [unwired: 2 in, 3 out]
                n501 = invoke on="インボークノード" class="List`1[[Konicaminolta.Lvxy, LC-" method="Add"(reference=w898, "item"=w899) -> (reference out=w906:refnum<k24>)  [unwired: 2 in, 3 out]
                n502 = invoke on="インボークノード" class="List`1[[Konicaminolta.Lvxy, LC-" method="Add"(reference=w906, "item"=w914) -> (reference out=w911:refnum<k24>)  [unwired: 2 in, 3 out]
                n503 = invoke on="インボークノード" class="List`1[[Konicaminolta.Lvxy, LC-" method="Add"(reference=w911, "item"=w912) -> (reference out=w909:refnum<k24>)  [unwired: 2 in, 3 out]
                n504 = invoke on="インボークノード" class="List`1[[Konicaminolta.Lvxy, LC-" method="Add"(reference=w909, "item"=w910) -> (reference out=w897:refnum<k24>)  [unwired: 2 in, 3 out]
                n505 = invoke on="インボークノード" class="List`1[[Konicaminolta.Lvxy, LC-" method="Add"(reference=w903, "item"=w902) -> (reference out=w908:refnum<k24>)  [unwired: 2 in, 3 out]
                n506 = invoke on="インボークノード" class="List`1[[Konicaminolta.Lvxy, LC-" method="Add"(reference=w908, "item"=w901) -> (reference out=w907:refnum<k24>)  [unwired: 2 in, 3 out]
                n507 = invoke on="インボークノード" class="List`1[[Konicaminolta.Lvxy, LC-" method="Add"(reference=w907, "item"=w900) -> (reference out=w896:refnum<k24>)  [unwired: 2 in, 3 out]
              }
            }
            n508 = invoke on="インボークノード" class="LightColorMISDK" method="SetMatrixCalib"(reference=w823, "calibrationCh"=w822, "measurementDataList"=w813, "correctDataList"=w812, "type"=w814, "id"=w821, "comPort"=0) -> (error out=w819:errorcluster, "SetMatrixCalib"=w820:refnum<k24>)  [unwired: 2 in, 7 out]
            n509 = property on="プロパティノード" class="ReturnMessage"(reference=w820, error in=w819) -> (error out=w818:errorcluster, "errorCode"=w811:i32)  [unwired: 1 out]
            n510 = property on="error out" class="Clust （指定）"("Value"=w818) -> ()  [unwired: 2 in, 2 out]
            n511 = property on="CalError" class="DigNum （指定）"("Value"=w811) -> ()  [unwired: 2 in, 2 out]
          }
        }
      }
      event "Calib.Ch": Value Change {
        n512 = event-data() -> ()  [unwired: 1 in, 6 out]
        n513 = case shown="\"U06\"" "Calib.Ch" {
          selector: "Calib.Ch" -> [w969 w972 w975 w978 w981 w984 w987 w990 w993 w996]
          tunnel: [w967 w970 w973 w976 w979 w982 w985 w988 w991 w994] -> w963
          frame "U01", Default {
            n514 = Add(x=w969, y=1) -> (x+y=w967:i32)
          }
          frame "U02" {
            n515 = Add(x=w972, y=1) -> (x+y=w970:i32)
          }
          frame "U03" {
            n516 = Add(x=w975, y=1) -> (x+y=w973:i32)
          }
          frame "U04" {
            n517 = Add(x=w978, y=1) -> (x+y=w976:i32)
          }
          frame "U05" {
            n518 = Add(x=w981, y=1) -> (x+y=w979:i32)
          }
          frame "U06" {
            n519 = Add(x=w984, y=1) -> (x+y=w982:i32)
          }
          frame "U07" {
            n520 = Add(x=w987, y=1) -> (x+y=w985:i32)
          }
          frame "U08" {
            n521 = Add(x=w990, y=1) -> (x+y=w988:i32)
          }
          frame "U09" {
            n522 = Add(x=w993, y=1) -> (x+y=w991:i32)
          }
          frame "U10" {
            n523 = Add(x=w996, y=1) -> (x+y=w994:i32)
          }
        }
        n524 = flat-sequence {
          tunnel: w966 -> [w1006]
          tunnel: [w1004] -> w965
          tunnel: w963 -> [w1002]
          tunnel: [w1000] -> w962
          tunnel: [w999] -> w961
          tunnel: [w998] -> w960
          tunnel: w965 -> [w1010]
          tunnel: w962 -> [w1009]
          tunnel: w961 -> [w1008]
          tunnel: w960 -> [w1007]
          frame #0 {
            n525 = invoke on="インボークノード" class="LightColorMISDK" method="GetCalibData"(reference=w1006, "calibrationCh"=w1002, "comPort"=0) -> ("GetCalibData"=w1003:refnum<k24>, "measurementDataList"=w1004:refnum<k24>, "correctDataList"=w998:refnum<k24>, "colorValueCalibrationData"=w999:refnum<k24>)  [unwired: 5 in, 4 out]
            n526 = property on="プロパティノード" class="ReturnMessage"(reference=w1003) -> ("errorCode"=w997:i32)  [unwired: 1 in, 2 out]
            "ErrorCode" <- w997
            n527 = Equal?(x=w997, y=0) -> (x = y?=w1000:bool)
          }
          frame #1 {
            n528 = case shown="TRUE" w1009 {
              tunnel: w1010 -> [_ w1029]
              tunnel: w1008 -> [_ w1028]
              tunnel: w1007 -> [_ w1013]
              frame False {
                n529 = property on="ID" class="Str"("Value"="") -> ()  [unwired: 2 in, 2 out]
              }
              frame True {
                n530 = control-ref of="After_B"() -> (w1023:refnum<vi>)
                n531 = control-ref of="After_G"() -> (w1021:refnum<vi>)
                n532 = control-ref of="After_W"() -> (w1014:refnum<vi>)
                n533 = control-ref of="After_R"() -> (w1019:refnum<vi>)
                n534 = control-ref of="Before_G"() -> (w1020:refnum<vi>)
                n535 = control-ref of="Before_G 2"() -> (w1017:refnum<vi>)
                n536 = control-ref of="Before_B 2"() -> (w1015:refnum<vi>)
                n537 = control-ref of="Before_W 2"() -> (w1024:refnum<vi>)
                n538 = control-ref of="Before_R 2"() -> (w1018:refnum<vi>)
                n539 = control-ref of="Before_W"() -> (w1025:refnum<vi>)
                n540 = property on="プロパティノード" class="UserCalibData"(reference=w1028) -> ("CalibType"=w1026:i32, "Id"=w1012:string)  [unwired: 1 in, 2 out]
                n541 = control-ref of="Before_R"() -> (w1016:refnum<vi>)
                n542 = case shown="0, デフォルト" w1026 {
                  tunnel: [1 3 4] -> w1027
                  frame 0, Default {
                  }
                  frame 1 {
                  }
                  frame 2 {
                  }
                }
                n543 = control-ref of="Before_B"() -> (w1022:refnum<vi>)
                n544 = property on="Type of Calibration" class="RadioBtnsControl （指定）"("Value"=w1026) -> ()  [unwired: 2 in, 2 out]
                n545 = property on="ID" class="Str"("Value"=w1012) -> ()  [unwired: 2 in, 2 out]
                n546 = call "LC-MISDK_UserCalibration_TypeofCalib.vi"("Cluster入力"=w1025, "Bool refnum 3"=w1017, "Clust refnum 4"=w1019, "Bool refnum 2"=w1018, "Clust refnum 5"=w1020, "Clust refnum 3"=w1016, "Clust refnum 6"=w1021, "Bool refnum 4"=w1015, "Clust refnum 7"=w1022, "Clust refnum入力"=w1014, "Clust refnum 8"=w1023, "Type of Calibration"=w1026, "Bool refnum"=w1024) -> ()  [unwired: 7 in]
                n547 = for {
                  N: w1027 -> [w1051]
                  tunnel: w1029 -> [w1055]
                  tunnel: w1013 -> [w1046]
                  i -> [w1044]
                  n548 = invoke on="インボークノード" class="List`1[[Konicaminolta.Measureme" method="get_Item"(reference=w1046, "index"=w1044) -> ("get_Item"=w1043:refnum<k24>)  [unwired: 2 in, 3 out]
                  n549 = invoke on="インボークノード" class="List`1[[Konicaminolta.Measureme" method="get_Item"(reference=w1055, "index"=w1044) -> (error out=w1053:errorcluster, "get_Item"=w1054:refnum<k24>)  [unwired: 2 in, 2 out]
                  n550 = property on="プロパティノード" class="MeasurementData"(reference=w1043) -> ("ColorSpaceValue"=w1042:refnum<k24>)  [unwired: 1 in, 2 out]
                  n551 = property on="プロパティノード" class="MeasurementData"(reference=w1054, error in=w1053) -> (error out=w1034:errorcluster, "ColorSpaceValue"=w1052:refnum<k24>, "ColorModeId"=w1045:i32)  [unwired: 1 out]
                  n552 = property on="Color Space" class="Enum （指定）"("Value"=w1045) -> ()  [unwired: 2 in, 2 out]
                  n553 = case shown="1" w1045 {
                    tunnel: ["y" "vd" "duv" "Z" "Pe"] -> w1039
                    tunnel: ["x" "ud" "Tcp" "Y" "λd"] -> w1040
                    tunnel: ["Lv" "Lv" "Lv" "X" "Lv"] -> w1041
                    frame 0, Default {
                    }
                    frame 1 {
                    }
                    frame 2 {
                    }
                    frame 3 {
                    }
                    frame 4 {
                    }
                  }
                  n554 = invoke class="Dictionary`2[[System.String, ms" method="get_Item"(reference=w1042, error in=w1034, "key"=w1041) -> ("get_Item"=w1038:dbl)  [unwired: 1 in, 3 out]
                  n555 = invoke class="Dictionary`2[[System.String, ms" method="get_Item"(reference=w1042, error in=w1034, "key"=w1039) -> (error out=→"error out":errorcluster, "get_Item"=w1036:dbl)  [unwired: 1 in, 2 out]
                  n556 = invoke class="Dictionary`2[[System.String, ms" method="get_Item"(reference=w1042, error in=w1034, "key"=w1040) -> ("get_Item"=w1037:dbl)  [unwired: 1 in, 3 out]
                  n557 = invoke on="インボークノード" class="Dictionary`2[[System.String, ms" method="get_Item"(reference=w1052, "key"=w1039) -> ("get_Item"=w1048:dbl)  [unwired: 2 in, 3 out]
                  n558 = invoke on="インボークノード" class="Dictionary`2[[System.String, ms" method="get_Item"(reference=w1052, "key"=w1041) -> ("get_Item"=w1050:dbl)  [unwired: 2 in, 3 out]
                  n559 = invoke on="インボークノード" class="Dictionary`2[[System.String, ms" method="get_Item"(reference=w1052, "key"=w1040) -> ("get_Item"=w1049:dbl)  [unwired: 2 in, 3 out]
                  n560 = Bundle("get_Item"=w1038, "get_Item"=w1037, "get_Item"=w1036) -> (w1035:T11)  [unwired: 1 in]
                  n561 = Bundle("get_Item"=w1050, "get_Item"=w1049, "get_Item"=w1048) -> (w1047:T11)  [unwired: 1 in]
                  n562 = case shown="1, デフォルト" w1051 {
                    tunnel: w1047 -> [w1217 w1220 w1229]
                    tunnel: w1044 -> [_ w1219 w1228]
                    tunnel: w1035 -> [w1216 w1218 w1227]
                    frame 1, Default {
                      n563 = property on="Before_W" class="Clust （指定）"("Value"=w1217) -> ()  [unwired: 2 in, 2 out]
                      n564 = property on="After_W" class="Clust （指定）"("Value"=w1216) -> ()  [unwired: 2 in, 2 out]
                    }
                    frame 3 {
                      n565 = case shown="1" w1219 {
                        tunnel: w1220 -> [w1222 w1224 w1226]
                        tunnel: w1218 -> [w1221 w1223 w1225]
                        frame 0, Default {
                          n566 = property on="Before_R" class="Clust （指定）"("Value"=w1222) -> ()  [unwired: 2 in, 2 out]
                          n567 = property on="After_R" class="Clust （指定）"("Value"=w1221) -> ()  [unwired: 2 in, 2 out]
                        }
                        frame 1 {
                          n568 = property on="Before_G" class="Clust （指定）"("Value"=w1224) -> ()  [unwired: 2 in, 2 out]
                          n569 = property on="After_G" class="Clust （指定）"("Value"=w1223) -> ()  [unwired: 2 in, 2 out]
                        }
                        frame 2 {
                          n570 = property on="Before_B" class="Clust （指定）"("Value"=w1226) -> ()  [unwired: 2 in, 2 out]
                          n571 = property on="After_B" class="Clust （指定）"("Value"=w1225) -> ()  [unwired: 2 in, 2 out]
                        }
                      }
                    }
                    frame 4 {
                      n572 = case shown="0, デフォルト" w1228 {
                        tunnel: w1229 -> [w1231 w1233 w1235 w1237]
                        tunnel: w1227 -> [w1230 w1232 w1234 w1236]
                        frame 0, Default {
                          n573 = property on="Before_W" class="Clust （指定）"("Value"=w1231) -> ()  [unwired: 2 in, 2 out]
                          n574 = property on="After_W" class="Clust （指定）"("Value"=w1230) -> ()  [unwired: 2 in, 2 out]
                        }
                        frame 1 {
                          n575 = property on="Before_R" class="Clust （指定）"("Value"=w1233) -> ()  [unwired: 2 in, 2 out]
                          n576 = property on="After_R" class="Clust （指定）"("Value"=w1232) -> ()  [unwired: 2 in, 2 out]
                        }
                        frame 2 {
                          n577 = property on="Before_G" class="Clust （指定）"("Value"=w1235) -> ()  [unwired: 2 in, 2 out]
                          n578 = property on="After_G" class="Clust （指定）"("Value"=w1234) -> ()  [unwired: 2 in, 2 out]
                        }
                        frame 3 {
                          n579 = property on="Before_B" class="Clust （指定）"("Value"=w1237) -> ()  [unwired: 2 in, 2 out]
                          n580 = property on="After_B" class="Clust （指定）"("Value"=w1236) -> ()  [unwired: 2 in, 2 out]
                        }
                      }
                    }
                  }
                  n581 = case shown="1" w1045 {
                    frame 0, Default {
                      w1059 = refnum<vi> refnum  # テキスト
                      w1064 = refnum<vi> refnum  # テキスト
                      w1067 = refnum<vi> refnum  # テキスト
                      w1074 = refnum<vi> refnum  # テキスト
                      w1079 = refnum<vi> refnum  # テキスト
                      w1084 = refnum<vi> refnum  # テキスト
                      n582 = property class="VI"() -> ("Panel"=w1087:refnum<vi>)  [unwired: 2 in, 2 out]
                      n583 = property class="Pnl"(reference=w1087) -> ("Decos[]"=w1056:refnum<vi>[])  [unwired: 1 in, 2 out]
                      n584 = Index Array(array=w1056, index=2) -> (element=w1086:refnum<vi>)
                      n585 = Index Array(array=w1056, index=17) -> (element=w1069:refnum<vi>)
                      n586 = Index Array(array=w1056, index=0) -> (element=w1076:refnum<vi>)
                      n587 = Index Array(array=w1056, index=1) -> (element=w1081:refnum<vi>)
                      n588 = Index Array(array=w1056, index=15) -> (element=w1061:refnum<vi>)
                      n589 = Index Array(array=w1056, index=16) -> (element=w1066:refnum<vi>)
                      n590 = To More Specific Class(target class=w1084, reference=w1086) -> (specific class reference=w1085:refnum<vi>)  [unwired: 1 in, 1 out]
                      n591 = To More Specific Class(target class=w1067, reference=w1069) -> (specific class reference=w1071:refnum<vi>)  [unwired: 1 in, 1 out]
                      n592 = To More Specific Class(target class=w1074, reference=w1076) -> (specific class reference=w1075:refnum<vi>)  [unwired: 1 in, 1 out]
                      n593 = To More Specific Class(target class=w1079, reference=w1081) -> (specific class reference=w1080:refnum<vi>)  [unwired: 1 in, 1 out]
                      n594 = To More Specific Class(target class=w1059, reference=w1061) -> (specific class reference=w1060:refnum<vi>)  [unwired: 1 in, 1 out]
                      n595 = To More Specific Class(target class=w1064, reference=w1066) -> (specific class reference=w1065:refnum<vi>)  [unwired: 1 in, 1 out]
                      n596 = property class="Txt"(reference=w1085, "Text"="Lv") -> ()  [unwired: 1 in, 2 out]
                      n597 = property class="Txt"(reference=w1071, "Text"="Lv") -> ()  [unwired: 1 in, 2 out]
                      n598 = property class="Txt"(reference=w1075, "Text"="y") -> ()  [unwired: 1 in, 2 out]
                      n599 = property class="Txt"(reference=w1080, "Text"="x") -> ()  [unwired: 1 in, 2 out]
                      n600 = property class="Txt"(reference=w1060, "Text"="y") -> ()  [unwired: 1 in, 2 out]
                      n601 = property class="Txt"(reference=w1065, "Text"="x") -> ()  [unwired: 1 in, 2 out]
                    }
                    frame 1 {
                      w1091 = refnum<vi> refnum  # テキスト
                      w1096 = refnum<vi> refnum  # テキスト
                      w1099 = refnum<vi> refnum  # テキスト
                      w1106 = refnum<vi> refnum  # テキスト
                      w1111 = refnum<vi> refnum  # テキスト
                      w1116 = refnum<vi> refnum  # テキスト
                      n602 = property class="VI"() -> ("Panel"=w1119:refnum<vi>)  [unwired: 2 in, 2 out]
                      n603 = property class="Pnl"(reference=w1119) -> ("Decos[]"=w1088:refnum<vi>[])  [unwired: 1 in, 2 out]
                      n604 = Index Array(array=w1088, index=2) -> (element=w1118:refnum<vi>)
                      n605 = Index Array(array=w1088, index=17) -> (element=w1101:refnum<vi>)
                      n606 = Index Array(array=w1088, index=0) -> (element=w1108:refnum<vi>)
                      n607 = Index Array(array=w1088, index=1) -> (element=w1113:refnum<vi>)
                      n608 = Index Array(array=w1088, index=15) -> (element=w1093:refnum<vi>)
                      n609 = Index Array(array=w1088, index=16) -> (element=w1098:refnum<vi>)
                      n610 = To More Specific Class(target class=w1116, reference=w1118) -> (specific class reference=w1117:refnum<vi>)  [unwired: 1 in, 1 out]
                      n611 = To More Specific Class(target class=w1099, reference=w1101) -> (specific class reference=w1103:refnum<vi>)  [unwired: 1 in, 1 out]
                      n612 = To More Specific Class(target class=w1106, reference=w1108) -> (specific class reference=w1107:refnum<vi>)  [unwired: 1 in, 1 out]
                      n613 = To More Specific Class(target class=w1111, reference=w1113) -> (specific class reference=w1112:refnum<vi>)  [unwired: 1 in, 1 out]
                      n614 = To More Specific Class(target class=w1091, reference=w1093) -> (specific class reference=w1092:refnum<vi>)  [unwired: 1 in, 1 out]
                      n615 = To More Specific Class(target class=w1096, reference=w1098) -> (specific class reference=w1097:refnum<vi>)  [unwired: 1 in, 1 out]
                      n616 = property class="Txt"(reference=w1117, "Text"="Lv") -> ()  [unwired: 1 in, 2 out]
                      n617 = property class="Txt"(reference=w1103, "Text"="Lv") -> ()  [unwired: 1 in, 2 out]
                      n618 = property class="Txt"(reference=w1107, "Text"="v") -> ()  [unwired: 1 in, 2 out]
                      n619 = property class="Txt"(reference=w1112, "Text"="u") -> ()  [unwired: 1 in, 2 out]
                      n620 = property class="Txt"(reference=w1092, "Text"="v") -> ()  [unwired: 1 in, 2 out]
                      n621 = property class="Txt"(reference=w1097, "Text"="u") -> ()  [unwired: 1 in, 2 out]
                    }
                    frame 2 {
                      w1123 = refnum<vi> refnum  # テキスト
                      w1128 = refnum<vi> refnum  # テキスト
                      w1131 = refnum<vi> refnum  # テキスト
                      w1138 = refnum<vi> refnum  # テキスト
                      w1143 = refnum<vi> refnum  # テキスト
                      w1148 = refnum<vi> refnum  # テキスト
                      n622 = property class="VI"() -> ("Panel"=w1151:refnum<vi>)  [unwired: 2 in, 2 out]
                      n623 = property class="Pnl"(reference=w1151) -> ("Decos[]"=w1120:refnum<vi>[])  [unwired: 1 in, 2 out]
                      n624 = Index Array(array=w1120, index=2) -> (element=w1150:refnum<vi>)
                      n625 = Index Array(array=w1120, index=17) -> (element=w1133:refnum<vi>)
                      n626 = Index Array(array=w1120, index=0) -> (element=w1140:refnum<vi>)
                      n627 = Index Array(array=w1120, index=1) -> (element=w1145:refnum<vi>)
                      n628 = Index Array(array=w1120, index=15) -> (element=w1125:refnum<vi>)
                      n629 = Index Array(array=w1120, index=16) -> (element=w1130:refnum<vi>)
                      n630 = To More Specific Class(target class=w1148, reference=w1150) -> (specific class reference=w1149:refnum<vi>)  [unwired: 1 in, 1 out]
                      n631 = To More Specific Class(target class=w1131, reference=w1133) -> (specific class reference=w1135:refnum<vi>)  [unwired: 1 in, 1 out]
                      n632 = To More Specific Class(target class=w1138, reference=w1140) -> (specific class reference=w1139:refnum<vi>)  [unwired: 1 in, 1 out]
                      n633 = To More Specific Class(target class=w1143, reference=w1145) -> (specific class reference=w1144:refnum<vi>)  [unwired: 1 in, 1 out]
                      n634 = To More Specific Class(target class=w1123, reference=w1125) -> (specific class reference=w1124:refnum<vi>)  [unwired: 1 in, 1 out]
                      n635 = To More Specific Class(target class=w1128, reference=w1130) -> (specific class reference=w1129:refnum<vi>)  [unwired: 1 in, 1 out]
                      n636 = property class="Txt"(reference=w1149, "Text"="Lv") -> ()  [unwired: 1 in, 2 out]
                      n637 = property class="Txt"(reference=w1135, "Text"="Lv") -> ()  [unwired: 1 in, 2 out]
                      n638 = property class="Txt"(reference=w1139, "Text"="duv") -> ()  [unwired: 1 in, 2 out]
                      n639 = property class="Txt"(reference=w1144, "Text"="Tcp") -> ()  [unwired: 1 in, 2 out]
                      n640 = property class="Txt"(reference=w1124, "Text"="duv") -> ()  [unwired: 1 in, 2 out]
                      n641 = property class="Txt"(reference=w1129, "Text"="Tcp") -> ()  [unwired: 1 in, 2 out]
                    }
                    frame 3 {
                      w1155 = refnum<vi> refnum  # テキスト
                      w1160 = refnum<vi> refnum  # テキスト
                      w1163 = refnum<vi> refnum  # テキスト
                      w1170 = refnum<vi> refnum  # テキスト
                      w1175 = refnum<vi> refnum  # テキスト
                      w1180 = refnum<vi> refnum  # テキスト
                      n642 = property class="VI"() -> ("Panel"=w1183:refnum<vi>)  [unwired: 2 in, 2 out]
                      n643 = property class="Pnl"(reference=w1183) -> ("Decos[]"=w1152:refnum<vi>[])  [unwired: 1 in, 2 out]
                      n644 = Index Array(array=w1152, index=2) -> (element=w1182:refnum<vi>)
                      n645 = Index Array(array=w1152, index=17) -> (element=w1165:refnum<vi>)
                      n646 = Index Array(array=w1152, index=0) -> (element=w1172:refnum<vi>)
                      n647 = Index Array(array=w1152, index=1) -> (element=w1177:refnum<vi>)
                      n648 = Index Array(array=w1152, index=15) -> (element=w1157:refnum<vi>)
                      n649 = Index Array(array=w1152, index=16) -> (element=w1162:refnum<vi>)
                      n650 = To More Specific Class(target class=w1180, reference=w1182) -> (specific class reference=w1181:refnum<vi>)  [unwired: 1 in, 1 out]
                      n651 = To More Specific Class(target class=w1163, reference=w1165) -> (specific class reference=w1167:refnum<vi>)  [unwired: 1 in, 1 out]
                      n652 = To More Specific Class(target class=w1170, reference=w1172) -> (specific class reference=w1171:refnum<vi>)  [unwired: 1 in, 1 out]
                      n653 = To More Specific Class(target class=w1175, reference=w1177) -> (specific class reference=w1176:refnum<vi>)  [unwired: 1 in, 1 out]
                      n654 = To More Specific Class(target class=w1155, reference=w1157) -> (specific class reference=w1156:refnum<vi>)  [unwired: 1 in, 1 out]
                      n655 = To More Specific Class(target class=w1160, reference=w1162) -> (specific class reference=w1161:refnum<vi>)  [unwired: 1 in, 1 out]
                      n656 = property class="Txt"(reference=w1181, "Text"="X") -> ()  [unwired: 1 in, 2 out]
                      n657 = property class="Txt"(reference=w1167, "Text"="X") -> ()  [unwired: 1 in, 2 out]
                      n658 = property class="Txt"(reference=w1171, "Text"="Z") -> ()  [unwired: 1 in, 2 out]
                      n659 = property class="Txt"(reference=w1176, "Text"="Y") -> ()  [unwired: 1 in, 2 out]
                      n660 = property class="Txt"(reference=w1156, "Text"="Z") -> ()  [unwired: 1 in, 2 out]
                      n661 = property class="Txt"(reference=w1161, "Text"="Y") -> ()  [unwired: 1 in, 2 out]
                    }
                    frame 4 {
                      w1187 = refnum<vi> refnum  # テキスト
                      w1192 = refnum<vi> refnum  # テキスト
                      w1195 = refnum<vi> refnum  # テキスト
                      w1202 = refnum<vi> refnum  # テキスト
                      w1207 = refnum<vi> refnum  # テキスト
                      w1212 = refnum<vi> refnum  # テキスト
                      n662 = property class="VI"() -> ("Panel"=w1215:refnum<vi>)  [unwired: 2 in, 2 out]
                      n663 = property class="Pnl"(reference=w1215) -> ("Decos[]"=w1184:refnum<vi>[])  [unwired: 1 in, 2 out]
                      n664 = Index Array(array=w1184, index=2) -> (element=w1214:refnum<vi>)
                      n665 = Index Array(array=w1184, index=17) -> (element=w1197:refnum<vi>)
                      n666 = Index Array(array=w1184, index=0) -> (element=w1204:refnum<vi>)
                      n667 = Index Array(array=w1184, index=1) -> (element=w1209:refnum<vi>)
                      n668 = Index Array(array=w1184, index=15) -> (element=w1189:refnum<vi>)
                      n669 = Index Array(array=w1184, index=16) -> (element=w1194:refnum<vi>)
                      n670 = To More Specific Class(target class=w1212, reference=w1214) -> (specific class reference=w1213:refnum<vi>)  [unwired: 1 in, 1 out]
                      n671 = To More Specific Class(target class=w1195, reference=w1197) -> (specific class reference=w1199:refnum<vi>)  [unwired: 1 in, 1 out]
                      n672 = To More Specific Class(target class=w1202, reference=w1204) -> (specific class reference=w1203:refnum<vi>)  [unwired: 1 in, 1 out]
                      n673 = To More Specific Class(target class=w1207, reference=w1209) -> (specific class reference=w1208:refnum<vi>)  [unwired: 1 in, 1 out]
                      n674 = To More Specific Class(target class=w1187, reference=w1189) -> (specific class reference=w1188:refnum<vi>)  [unwired: 1 in, 1 out]
                      n675 = To More Specific Class(target class=w1192, reference=w1194) -> (specific class reference=w1193:refnum<vi>)  [unwired: 1 in, 1 out]
                      n676 = property class="Txt"(reference=w1213, "Text"="Lv") -> ()  [unwired: 1 in, 2 out]
                      n677 = property class="Txt"(reference=w1199, "Text"="Lv") -> ()  [unwired: 1 in, 2 out]
                      n678 = property class="Txt"(reference=w1203, "Text"="Pe") -> ()  [unwired: 1 in, 2 out]
                      n679 = property class="Txt"(reference=w1208, "Text"="λd") -> ()  [unwired: 1 in, 2 out]
                      n680 = property class="Txt"(reference=w1188, "Text"="Pe") -> ()  [unwired: 1 in, 2 out]
                      n681 = property class="Txt"(reference=w1193, "Text"="λd") -> ()  [unwired: 1 in, 2 out]
                    }
                  }
                }
              }
            }
          }
        }
      }
    }
  }
